vi "5.0.4_HH_Restriction.vi"(6 "Data in":T1, 8 "error in (no error)":errorcluster, 9 "AllControls In":T2, 10 "?":T3, 11 "Message Queue out":T4) -> (0 "error out":errorcluster, 1 "Flow":string, 2 "Data":T3, 3 "Message Queue Out":T4, 4 "Data out":T1)   [LabVIEW 2017]
uses:
  Depends/AMC/subVIs/TypeDefs/amc_Message Queue.ctl
  Depends/AMC/subVIs/TypeDefs/amc_Message.ctl
  Depends/Tools/Keyed Array/Tools_KeyedArray KeyedArray.ctl
  Ctrls/Data.ctl
  Ctrls/AllControls.ctl
  Ctrls/CSV_Data.ctl
  DIPC 692 Daemon API/typdef/get_parameter.ctl
  DIPC 692 Daemon API/typdef/task_detect_test_point.ctl
  DIPC 692 Daemon API/typdef/calibration.ctl
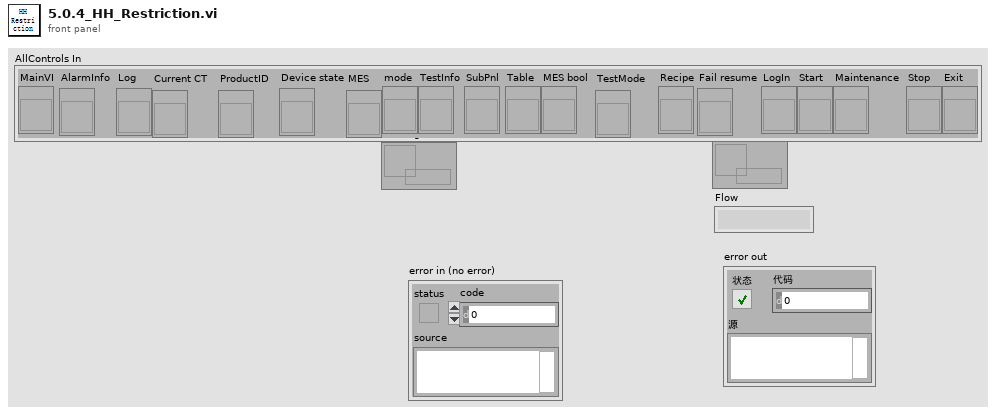
[diagram p1: front panel]
types:
  T1 = typedef "CSV_Data.ctl" = cluster{"Initialisation":cluster{"LMT - Connect UUT (con COM)":string, "LMT - Software Version (rrel)":string, "LMT - Write SKU file (wskuc)":string, "LMT - SKU file name":string, "Connect UUT DDM":string, "Read DDM EOL Timestamp - Mode":string, "Read DDM EOL Timestamp - Timestamp":string, "Read DDM EOL Timestamp - Rig ID":string, "Read DDM EOL Timestamp - Passmark ID":string, "Read DDM EOL Timestamp - Passmark Rev":string, "Software Version before flashing":string, "Read Hardware Serial":string, "UUT DDM SN":string, "Compare DDM SN with MES SN":string, "Backup PCBA Calibration EEPROM Response - CAL":string, "Flash Firmware Version":string, "Check SW Version":string, "Read DDM SW Version after flashing":string, "Set SKU Config":string, "Ready Status":string, "Set Device Mode to EOL":string, "DDM Parameter - Voltage":string, "DDM Parameter - Current":string, "DDM Parameter - Power":string, "DDM Parameter - Speed":string, "DDM Parameter - Pressure":string, "Tester Parameter - Voltage":string, "Tester Parameter - Current":string, "Tester Parameter - Power":string, "Tester Parameter - Ambient Pressure":string, "Tester Parameter - Ambient Temperature":string, "Calculated Parameter - DDM Pressure Corrected":string, "Calculated Parameter - DDM Real Power":string, "Calculated Parameter - Delta V":string}, "BEMF_Calibration":cluster{"Calibration Result - eol_cold_bemf_temp":string, "DDM Ambient Temp":string, "Restriction Plate Diameter":string, "Calibration Result - eol_bemf_mp_cold_coef_a":string, "Calibration Result - eol_bemf_mp_cold_coef_b":string, "Calibration Result - eol_bemf_mp_cold_coef_c":string, "Calibration Result - eol_bemf_lsi_cold_ref_coeffs":string, "Get - Calibration Result - eol_bemf_lsi_speed":string, "Get - Calibration Result - eol_bemf_lsi_integral_0":string, "Calibration Result - eol_bemf_lsi_integral_1":string, "Get - Calibration Result - eol_bemf_lsi_integral_2":string, "Get - Calibration Result - eol_cold_bemf":string, "Get - Calibration Result - eol_cold_bemf_fisf":string, "Finalise Calibration":string, "Compare -Calibration Result - eol_cold_bemf":string, "Compare -Calibration Result - eol_cold_bemf_fisf":string}, "ECO":cluster{"Reset Power Tune":string, "Reset BEMF FISF Calibration":string, "Restriction Plate Diameter":string, "ECO - Stabilisation Time":string, "ECO - DDM Parameter - Voltage":string, "ECO - DDM Parameter - Current":string, "ECO - DDM Parameter - Power":string, "ECO - DDM Parameter - Measured Power":string, "ECO - DDM Parameter - Speed":string, "ECO - DDM Parameter - Pressure":string, "ECO - Tester Parameter - Voltage":string, "ECO - Tester Parameter - Current":string, "ECO - Tester Parameter - Power":string, "ECO - Tester Parameter - Ambient Pressure":string, "ECO - Tester Parameter - Ambient Temperature":string, "ECO - Tester Parameter - Ambient Humidity":string, "ECO - Calculated Parameter - DDM Pressure Corrected":string, "ECO - Calculated Parameter - DDM Real Power":string, "ECO - Calculated Parameter - Delta V":string, "ECO - Calculated Parameter - Flowrate":string, "ECO - Calculated Parameter - Airwatt":string, "ECO - Formula":string, "PT ECO - Power Tune Mode Status":string}, "BOOST":cluster{"Restriction Plate Diameter":string, "BOOST - Stabilisation Time":string, "BOOST - DDM Parameter - Voltage":string, "BOOST - DDM Parameter - Current":string, "BOOST - DDM Parameter - Power":string, "BOOST - DDM Parameter - Measured Power":string, "BOOST - DDM Parameter - Speed":string, "BOOST - DDM Parameter - Pressure":string, "BOOST - Tester Parameter - Voltage":string, "BOOST - Tester Parameter - Current":string, "BOOST - Tester Parameter - Power":string, "BOOST - Tester Parameter - Ambient Pressure":string, "BOOST - Tester Parameter - Ambient Temperature":string, "BOOST - Tester Parameter - Ambient Humidity":string, "BOOST - Calculated Parameter - DDM Pressure Corrected":string, "BOOST - Calculated Parameter - DDM Real Power":string, "BOOST - Calculated Parameter - Delta V":string, "BOOST - Calculated Parameter - Flowrate":string, "BOOST - Calculated Parameter - Airwatt":string, "BOOST - Get AM Presence":string, "Air Muscle Turn Off Status":string, "BOOST - Air Muscle Calculated Parameter - Airwatt B":string, "BOOST - Air Muscle Calculate Airwatt Delta":string, "PT BOOST - Power Tune Mode Status":string, "Finalise Calibration":string, "ECO - Get AW Calibration value":string, "BOOST - Get AW Calibration value":string}, "MAX":cluster{"Restriction Plate Diameter":string, "MAX - Stabilisation Time":string, "Get Average Delta Tmag (LSIdelta_FISFdelta_LSItmag_FISFtmag_IIRtmag)":string, "Get Average Delta Tmag FISF":string, "MAX - DDM Parameter - Voltage":string, "MAX - DDM Parameter - Current":string, "MAX - DDM Parameter - Power":string, "MAX - DDM Parameter - Measured Power":string, "MAX - DDM Parameter - Speed":string, "MAX - DDM Parameter - Pressure":string, "MAX - Tester Parameter - Voltage":string, "MAX - Tester Parameter - Current":string, "MAX - Tester Parameter - Power":string, "MAX - Tester Parameter - Ambient Pressure":string, "MAX - Tester Parameter - Ambient Temperature":string, "MAX - Tester Parameter - Ambient Humidity":string, "MAX - Calculated Parameter - DDM Pressure Corrected":string, "MAX - Calculated Parameter - DDM Real Power":string, "MAX - Calculated Parameter - Delta V":string, "MAX - Calculated Parameter - Flowrate":string, "MAX - Calculated Parameter - Airwatt":string, "MAX_FISF_Check_Average_Delta_Tmag":string, "MAX - FISF - BEMF Finetune Result":string, "MAX tune - Delta P1":string, "MAX tune - Calculated Parameter - Airwatt":string, "Calculate Delta Airwatts - MAX finetune - Delta P2":string, "MAX finetune - DDM Parameter - Voltage":string, "MAX finetune - DDM Parameter - Current":string, "MAX finetune - DDM Parameter - Power":string, "MAX finetune - DDM Parameter - Measured Power":string, "MAX finetune - DDM Parameter - Speed":string, "MAX finetune - DDM Parameter - Pressure":string, "MAX finetune - Tester Parameter - Voltage":string, "MAX finetune - Tester Parameter - Current":string, "MAX finetune - Tester Parameter - Power":string, "MAX finetune - Tester Parameter - Ambient Pressure":string, "MAX finetune - Tester Parameter - Ambient Temperature":string, "MAX finetune - Tester Parameter - Ambient Humidity":string, "MAX finetune - Calculated Parameter - DDM Pressure Corrected":string, "MAX finetune - Calculated Parameter - DDM Real Power":string, "MAX finetune - Calculated Parameter - Delta V":string, "MAX finetune - Calculated Parameter - Flowrate":string, "MAX finetune - Calculated Parameter - Airwatt":string, "Check Derate Result":string, "Delta Tmag FISF":string, "Get Hot BEMF Result":string, "Calculate delta Pressure":string, "Finalise Calibration":string, "Calculate & Check Delta BEMF":string, "Delta P Airwatts Value":string}, "LL":cluster{"DDM Ambient Temp":string, "Restriction Plate Diameter":string, "LL - DDM Parameter - Voltage":string, "LL - DDM Parameter - Current":string, "LL - DDM Parameter - Power":string, "LL - DDM Parameter - Measured Power":string, "LL - DDM Parameter - Speed":string, "LL - DDM Parameter - Pressure":string, "LL - Tester Parameter - Voltage":string, "LL - Tester Parameter - Current":string, "LL - Tester Parameter - Power":string, "LL - DDM Real Power":string, "LL - Calibrate Task Detect LL":string}, "HL":cluster{"HL - DDM Parameter - Voltage":string, "HL - DDM Parameter - Current":string, "HL - DDM Parameter - Power":string, "HL - DDM Parameter - Measured Power":string, "HL - DDM Parameter - Speed":string, "HL - DDM Parameter - Pressure":string, "HL - Tester Parameter - Voltage":string, "HL - Tester Parameter - Current":string, "HL - Tester Parameter - Power":string, "HL - DDM Real Power":string, "HL - Calibrate Task Detect HL":string}, "LH":cluster{"Restriction Plate Diameter":string, "LH - DDM Parameter - Voltage":string, "LH - DDM Parameter - Current":string, "LH - DDM Parameter - Power":string, "LH - DDM Parameter - Measured Power":string, "LH - DDM Parameter - Speed":string, "LH - DDM Parameter - Pressure":string, "LH - Tester Parameter - Voltage":string, "LH - Tester Parameter - Current":string, "LH - Tester Parameter - Power":string, "LH - DDM Real Power":string, "LH - Calibrate Task Detect LH":string}, "HH":cluster{"HH - DDM Parameter - Voltage":string, "HH - DDM Parameter - Current":string, "HH - DDM Parameter - Power":string, "HH - DDM Parameter - Measured Power":string, "HH - DDM Parameter - Speed":string, "HH - DDM Parameter - Pressure":string, "HH - Tester Parameter - Voltage":string, "HH - Tester Parameter - Current":string, "HH - Tester Parameter - Power":string, "HH - DDM Real Power":string, "HH - Calibrate Task Detect HH":string}, "Inlet Blockage Calibration":cluster{"Inlet Blockage Calibration - DDM Parameter - Voltage":string, "Inlet Blockage Calibration - DDM Parameter - Current":string, "Inlet Blockage Calibration - DDM Parameter - Power":string, "Inlet Blockage Calibration - DDM Parameter - Measured Power":string, "Inlet Blockage Calibration - DDM Parameter - Speed":string, "Inlet Blockage Calibration - DDM Parameter - Pressure":string, "Inlet Blockage Calibration - Tester Parameter - Voltage":string, "Inlet Blockage Calibration - Tester Parameter - Current":string, "Inlet Blockage Calibration - Tester Parameter - Power":string, "Inlet Blockage Calibration - DDM Real Power":string, "Calibration Inlet Blockage_E":string, "Finalise Calibration":string, "Get Task Detect LL":string, "Get Task Detect HL":string, "Get Task Detect LH":string, "Get Task Detect HH":string, "Calibration Inlet Blockage":string, "Calibration eol cold bemf temp":string}, "GOOD":cluster{"GOOD UNIT - Clear EEPROM Error Log":string, "GOOD UNIT - Write Product Timestamp - Mode":string, "GOOD UNIT - Write Product Timestamp - Timestamp":string, "GOOD UNIT - Write Product Timestamp - Rig ID":string, "GOOD UNIT - Write Product Timestamp - Passmark ID":string, "GOOD UNIT - Write Product Timestamp - Passmark Rev":string, "GOOD UNIT - Set Device Mode to PROD":string, "GOOD UNIT - Backup PCBA Calibration EEPROM Response":string, "GOOD UNIT - Check Security Bit":string, "GOOD UNIT - Set Calibration Lock":string, "GOOD UNIT - Get_Calibration_Lock":string, "GOOD UNIT - Disconnect UUT":string}, "NG":cluster{"NG UNIT - Read NVM Error":string, "NG UNIT - Set Device Mode to FCT":string, "NG UNIT - Backup PCBA Calibration EEPROM Response - CAL":string, "NG UNIT - Backup PCBA Calibration EEPROM Response - ERROR":string, "NG UNIT - Backup PCBA Calibration EEPROM Response - USAGE":string, "NG UNIT - Disconnect UUT":string}, "SN":string, "Table":string[][], "Count":cluster{"Total":i32, "OK":i32, "NG":i32, "Yield":dbl}, "Start Time":timestamp, "daemon reference":refnum<k5>, "CT":dbl, "Config":string[][], "OK/NG":bool, "Station ID":string, "MES DDM SN":string, "MES PCBA SN":string, "Retest":string, "Lux":string, "Initialisation_Status":cluster{"LMT - Connect UUT (con COM)":string, "LMT - Software Version (rrel)":string, "LMT - Write SKU file (wskuc)":string, "LMT - SKU file name":string, "Connect UUT DDM":string, "Read DDM EOL Timestamp - Mode":string, "Read DDM EOL Timestamp - Timestamp":string, "Read DDM EOL Timestamp - Rig ID":string, "Read DDM EOL Timestamp - Passmark ID":string, "Read DDM EOL Timestamp - Passmark Rev":string, "Software Version before flashing":string, "Read Hardware Serial":string, "UUT DDM SN":string, "Compare DDM SN with MES SN":string, "Backup PCBA Calibration EEPROM Response - CAL":string, "Flash Firmware Version":string, "Check SW Version":string, "Read DDM SW Version after flashing":string, "Set SKU Config":string, "Ready Status":string, "Set Device Mode to EOL":string, "DDM Parameter - Voltage":string, "DDM Parameter - Current":string, "DDM Parameter - Power":string, "DDM Parameter - Speed":string, "DDM Parameter - Pressure":string, "Tester Parameter - Voltage":string, "Tester Parameter - Current":string, "Tester Parameter - Power":string, "Tester Parameter - Ambient Pressure":string, "Tester Parameter - Ambient Temperature":string, "Calculated Parameter - DDM Pressure Corrected":string, "Calculated Parameter - DDM Real Power":string, "Calculated Parameter - Delta V":string}, "BEMF_Calibration_Status":cluster{"Calibration Result - eol_cold_bemf_temp":string, "DDM Ambient Temp":string, "Restriction Plate Diameter":string, "Calibration Result - eol_bemf_mp_cold_coef_a":string, "Calibration Result - eol_bemf_mp_cold_coef_b":string, "Calibration Result - eol_bemf_mp_cold_coef_c":string, "Calibration Result - eol_bemf_lsi_cold_ref_coeffs":string, "Get - Calibration Result - eol_bemf_lsi_speed":string, "Get - Calibration Result - eol_bemf_lsi_integral_0":string, "Calibration Result - eol_bemf_lsi_integral_1":string, "Get - Calibration Result - eol_bemf_lsi_integral_2":string, "Get - Calibration Result - eol_cold_bemf":string, "Get - Calibration Result - eol_cold_bemf_fisf":string, "Finalise Calibration":string, "Compare -Calibration Result - eol_cold_bemf":string, "Compare -Calibration Result - eol_cold_bemf_fisf":string}, "ECO_Status":cluster{"Reset Power Tune":string, "Reset BEMF FISF Calibration":string, "Restriction Plate Diameter":string, "ECO - Stabilisation Time":string, "ECO - DDM Parameter - Voltage":string, "ECO - DDM Parameter - Current":string, "ECO - DDM Parameter - Power":string, "ECO - DDM Parameter - Measured Power":string, "ECO - DDM Parameter - Speed":string, "ECO - DDM Parameter - Pressure":string, "ECO - Tester Parameter - Voltage":string, "ECO - Tester Parameter - Current":string, "ECO - Tester Parameter - Power":string, "ECO - Tester Parameter - Ambient Pressure":string, "ECO - Tester Parameter - Ambient Temperature":string, "ECO - Tester Parameter - Ambient Humidity":string, "ECO - Calculated Parameter - DDM Pressure Corrected":string, "ECO - Calculated Parameter - DDM Real Power":string, "ECO - Calculated Parameter - Delta V":string, "ECO - Calculated Parameter - Flowrate":string, "ECO - Calculated Parameter - Airwatt":string, "ECO - Formula":string, "PT ECO - Power Tune Mode Status":string}, "BOOST_Status":cluster{"Restriction Plate Diameter":string, "BOOST - Stabilisation Time":string, "BOOST - DDM Parameter - Voltage":string, "BOOST - DDM Parameter - Current":string, "BOOST - DDM Parameter - Power":string, "BOOST - DDM Parameter - Measured Power":string, "BOOST - DDM Parameter - Speed":string, "BOOST - DDM Parameter - Pressure":string, "BOOST - Tester Parameter - Voltage":string, "BOOST - Tester Parameter - Current":string, "BOOST - Tester Parameter - Power":string, "BOOST - Tester Parameter - Ambient Pressure":string, "BOOST - Tester Parameter - Ambient Temperature":string, "BOOST - Tester Parameter - Ambient Humidity":string, "BOOST - Calculated Parameter - DDM Pressure Corrected":string, "BOOST - Calculated Parameter - DDM Real Power":string, "BOOST - Calculated Parameter - Delta V":string, "BOOST - Calculated Parameter - Flowrate":string, "BOOST - Calculated Parameter - Airwatt":string, "BOOST - Get AM Presence":string, "Air Muscle Turn Off Status":string, "BOOST - Air Muscle Calculated Parameter - Airwatt B":string, "BOOST - Air Muscle Calculate Airwatt Delta":string, "PT BOOST - Power Tune Mode Status":string, "Finalise Calibration":string, "ECO - Get AW Calibration value":string, "BOOST - Get AW Calibration value":string}, "MAX_Status":cluster{"Restriction Plate Diameter":string, "MAX - Stabilisation Time":string, "Get Average Delta Tmag (LSIdelta_FISFdelta_LSItmag_FISFtmag_IIRtmag)":string, "Get Average Delta Tmag FISF":string, "MAX - DDM Parameter - Voltage":string, "MAX - DDM Parameter - Current":string, "MAX - DDM Parameter - Power":string, "MAX - DDM Parameter - Measured Power":string, "MAX - DDM Parameter - Speed":string, "MAX - DDM Parameter - Pressure":string, "MAX - Tester Parameter - Voltage":string, "MAX - Tester Parameter - Current":string, "MAX - Tester Parameter - Power":string, "MAX - Tester Parameter - Ambient Pressure":string, "MAX - Tester Parameter - Ambient Temperature":string, "MAX - Tester Parameter - Ambient Humidity":string, "MAX - Calculated Parameter - DDM Pressure Corrected":string, "MAX - Calculated Parameter - DDM Real Power":string, "MAX - Calculated Parameter - Delta V":string, "MAX - Calculated Parameter - Flowrate":string, "MAX - Calculated Parameter - Airwatt":string, "MAX_FISF_Check_Average_Delta_Tmag":string, "MAX - FISF - BEMF Finetune Result":string, "MAX tune - Delta P1":string, "MAX tune - Calculated Parameter - Airwatt":string, "Calculate Delta Airwatts - MAX finetune - Delta P2":string, "MAX finetune - DDM Parameter - Voltage":string, "MAX finetune - DDM Parameter - Current":string, "MAX finetune - DDM Parameter - Power":string, "MAX finetune - DDM Parameter - Measured Power":string, "MAX finetune - DDM Parameter - Speed":string, "MAX finetune - DDM Parameter - Pressure":string, "MAX finetune - Tester Parameter - Voltage":string, "MAX finetune - Tester Parameter - Current":string, "MAX finetune - Tester Parameter - Power":string, "MAX finetune - Tester Parameter - Ambient Pressure":string, "MAX finetune - Tester Parameter - Ambient Temperature":string, "MAX finetune - Tester Parameter - Ambient Humidity":string, "MAX finetune - Calculated Parameter - DDM Pressure Corrected":string, "MAX finetune - Calculated Parameter - DDM Real Power":string, "MAX finetune - Calculated Parameter - Delta V":string, "MAX finetune - Calculated Parameter - Flowrate":string, "MAX finetune - Calculated Parameter - Airwatt":string, "Check Derate Result":string, "Delta Tmag FISF":string, "Get Hot BEMF Result":string, "Calculate delta Pressure":string, "Finalise Calibration":string, "Calculate & Check Delta BEMF":string, "Delta P Airwatts Value":string}, "LL_Status":cluster{"DDM Ambient Temp":string, "Restriction Plate Diameter":string, "LL - DDM Parameter - Voltage":string, "LL - DDM Parameter - Current":string, "LL - DDM Parameter - Power":string, "LL - DDM Parameter - Measured Power":string, "LL - DDM Parameter - Speed":string, "LL - DDM Parameter - Pressure":string, "LL - Tester Parameter - Voltage":string, "LL - Tester Parameter - Current":string, "LL - Tester Parameter - Power":string, "LL - DDM Real Power":string, "LL - Calibrate Task Detect LL":string}, "HL_Status":cluster{"HL - DDM Parameter - Voltage":string, "HL - DDM Parameter - Current":string, "HL - DDM Parameter - Power":string, "HL - DDM Parameter - Measured Power":string, "HL - DDM Parameter - Speed":string, "HL - DDM Parameter - Pressure":string, "HL - Tester Parameter - Voltage":string, "HL - Tester Parameter - Current":string, "HL - Tester Parameter - Power":string, "HL - DDM Real Power":string, "HL - Calibrate Task Detect HL":string}, "LH_Status":cluster{"Restriction Plate Diameter":string, "LH - DDM Parameter - Voltage":string, "LH - DDM Parameter - Current":string, "LH - DDM Parameter - Power":string, "LH - DDM Parameter - Measured Power":string, "LH - DDM Parameter - Speed":string, "LH - DDM Parameter - Pressure":string, "LH - Tester Parameter - Voltage":string, "LH - Tester Parameter - Current":string, "LH - Tester Parameter - Power":string, "LH - DDM Real Power":string, "LH - Calibrate Task Detect LH":string}, "HH_Status":cluster{"HH - DDM Parameter - Voltage":string, "HH - DDM Parameter - Current":string, "HH - DDM Parameter - Power":string, "HH - DDM Parameter - Measured Power":string, "HH - DDM Parameter - Speed":string, "HH - DDM Parameter - Pressure":string, "HH - Tester Parameter - Voltage":string, "HH - Tester Parameter - Current":string, "HH - Tester Parameter - Power":string, "HH - DDM Real Power":string, "HH - Calibrate Task Detect HH":string}, "Inlet Blockage Calibration_Status":cluster{"Inlet Blockage Calibration - DDM Parameter - Voltage":string, "Inlet Blockage Calibration - DDM Parameter - Current":string, "Inlet Blockage Calibration - DDM Parameter - Power":string, "Inlet Blockage Calibration - DDM Parameter - Measured Power":string, "Inlet Blockage Calibration - DDM Parameter - Speed":string, "Inlet Blockage Calibration - DDM Parameter - Pressure":string, "Inlet Blockage Calibration - Tester Parameter - Voltage":string, "Inlet Blockage Calibration - Tester Parameter - Current":string, "Inlet Blockage Calibration - Tester Parameter - Power":string, "Inlet Blockage Calibration - DDM Real Power":string, "Calibration Inlet Blockage_E":string, "Finalise Calibration":string, "Get Task Detect LL":string, "Get Task Detect HL":string, "Get Task Detect LH":string, "Get Task Detect HH":string, "Calibration Inlet Blockage":string, "Calibration eol cold bemf temp":string}, "GOOD_Status":cluster{"GOOD UNIT - Clear EEPROM Error Log":string, "GOOD UNIT - Write Product Timestamp - Mode":string, "GOOD UNIT - Write Product Timestamp - Timestamp":string, "GOOD UNIT - Write Product Timestamp - Rig ID":string, "GOOD UNIT - Write Product Timestamp - Passmark ID":string, "GOOD UNIT - Write Product Timestamp - Passmark Rev":string, "GOOD UNIT - Set Device Mode to PROD":string, "GOOD UNIT - Backup PCBA Calibration EEPROM Response":string, "GOOD UNIT - Check Security Bit":string, "GOOD UNIT - Set Calibration Lock":string, "GOOD UNIT - Get_Calibration_Lock":string, "GOOD UNIT - Disconnect UUT":string}, "NG_Status":cluster{"NG UNIT - Read NVM Error":string, "NG UNIT - Set Device Mode to FCT":string, "NG UNIT - Backup PCBA Calibration EEPROM Response - CAL":string, "NG UNIT - Backup PCBA Calibration EEPROM Response - ERROR":string, "NG UNIT - Backup PCBA Calibration EEPROM Response - USAGE":string, "NG UNIT - Disconnect UUT":string}, "SKU":string, "Plate_Diameter":string, "Alarm":string}
  T2 = typedef "AllControls.ctl" = cluster{"MainVI":refnum<vi>, "AlarmInfo":refnum<vi>, "Log":refnum<vi>, "Current CT":refnum<vi>, "ProductID":refnum<vi>, "Device state":refnum<vi>, "MES":refnum<vi>, "mode":refnum<vi>, "TestInfo":refnum<vi>, "SubPnl":refnum<vi>, "Table":refnum<vi>, "MES bool":refnum<vi>, "TestMode":refnum<vi>, "Recipe":refnum<vi>, "Fail resume":refnum<vi>, "LogIn":refnum<vi>, "Start":refnum<vi>, "Maintenance":refnum<vi>, "Stop":refnum<vi>, "Exit":refnum<vi>}
  T3 = typedef "Data.ctl" = cluster{"Initialisation":cluster{"DDM_Parameter":dbl[], "DDM_Parameter_status":bool[], "Get_Tester_Parameter":dbl[], "Get_Tester_Parameter_status":bool[], "Cal_Tester_Parameter":dbl[], "Cal_Tester_Parameter_status":bool[], "sw_version_before_status":bool, "sw_version_after_status":bool, "Set_SKU_Config_With_LMT_status":bool, "FCT_timestamp_status":bool, "LMT_Connect_to_UUT_status":bool}, "BEMF_Calibration":cluster{"Read_ambient_temperature":dbl, "Calibration_Vaule":dbl[], "Calibration_Vaule _B":dbl[], "Calibration_Vaule_status":bool[], "Calibration_Vaule_B_status":bool[]}, "ECO":cluster{"DDM_Parameter":dbl[], "DDM_Parameter_status":bool[], "Get_Tester_Parameter":dbl[], "Get_Tester_Parameter_status":bool[], "Cal_Tester_Parameter":dbl[], "Cal_Tester_Parameter_status":bool[], "DDM_Parameter_after_power_tune":dbl[], "Get_Tester_Parameter_after_power_tune":dbl[], "Cal_Tester_Parameter_after_power_tune":dbl[], "Cal_Tester_Parameter_after_power_tune_status":bool[], "Delta_P":dbl}, "BOOST":cluster{"DDM_Parameter":dbl[], "DDM_Parameter_status":bool[], "Get_Tester_Parameter":dbl[], "Get_Tester_Parameter_status":bool[], "Cal_Tester_Parameter":dbl[], "Cal_Tester_Parameter_status":bool[], "DDM_Parameter_after_power_tune":dbl[], "Get_Tester_Parameter_after_power_tune":dbl[], "Cal_Tester_Parameter_after_power_tune":dbl[], "Cal_Tester_Parameter_after_power_tune_status":bool[], "airwatts_am_off":dbl, "AW_Delta_(AM_on_and_off)":dbl, "AW_Delta_(AM_on_and_off)_Status":bool, "Delta_P":dbl}, "MAX":cluster{"Average_Tmag_Data":cluster{"LSI Delta in degC":dbl, "FISF Delta in degc":dbl, "LSI Tmag in degC":dbl, "Fisf Tmag in degC":dbl, "IIR Tmag in degC":dbl}, "DDM_Parameter":dbl[], "DDM_Parameter_status":bool[], "Get_Tester_Parameter":dbl[], "Get_Tester_Parameter_status":bool[], "Cal_Tester_Parameter":dbl[], "BEMF_Finetune":cluster{"eol_bemf_mp_cold_coef_c":dbl, "eol_cold_bemf_fisf_offset":dbl}, "AW_Tune":cluster{"delta_P1":dbl, "delta_P_Setting":dbl}, "DDM_Parameter_after_Airwatts_Tune":dbl[], "Get_Tester_Parameter_after_Airwatts_Tune":dbl[], "Cal_Tester_Parameter_after_Airwatts_Tune":dbl[], "DDM_Parameter_after_Airwatts_Finetune":dbl[], "Get_Tester_Parameter_after_Airwatts_Finetune":dbl[], "Cal_Tester_Parameter_after_Airwatts_Finetune":dbl[], "AW_Finetune":cluster{"delta_P2":dbl, "delta_P_Setting":dbl}, "Delta_Tmag_after_tune":cluster{"LSI Delta in degC":dbl, "FISF Delta in degc":dbl, "LSI Tmag in degC":dbl, "Fisf Tmag in degC":dbl, "IIR Tmag in degC":dbl}, "Hot Bemf in mV":dbl, "DDM_Pressure":dbl, "Delta_Pressure":dbl, " Cold Bemf in mV":dbl, " delta Bemf":dbl, " delta p":dbl, "Delta_Pressure_status":bool, " delta Bemf_status":bool, "LSI Delta in degC_status":bool, "FISF Delta in degc_status":bool, "Max_check_derate_status_status":bool, "Average_All_data":dbl[][], "Average_Tmag_Data_status":bool[], "Average_Tmag_Data_after_tune_status":bool[], "Cal_Tester_Parameter_status":bool[], "Cal_Tester_Parameter_status_after_Airwatts_Tune":bool[], "Cal_Tester_Parameter_status_after_Airwatts_FineTune":bool[]}, "Task_Detect_Calib":cluster{"LL":cluster{"DDM_Parameter":dbl[], "DDM_Parameter_status":bool[], "Get_Tester_Parameter":dbl[], "Get_Tester_Parameter_status":bool[], "Set_task_detect_A":dbl, "Set_task_detect_A_Status":bool}, "HL":cluster{"DDM_Parameter":dbl[], "DDM_Parameter_status":bool[], "Get_Tester_Parameter":dbl[], "Get_Tester_Parameter_status":bool[], "Set_task_detect_B":dbl, "Set_task_detect_B_Status":bool}, "LH":cluster{"DDM_Parameter":dbl[], "DDM_Parameter_status":bool[], "Get_Tester_Parameter":dbl[], "Get_Tester_Parameter_status":bool[], "Set_task_detect_C":dbl, "Set_task_detect_C_Status":bool}, "HH":cluster{"DDM_Parameter":dbl[], "DDM_Parameter_status":bool[], "Get_Tester_Parameter":dbl[], "Get_Tester_Parameter_status":bool[], "Set_task_detect_D":dbl, "Read_and_check_calibration_Status":bool[], "Set_task_detect_D_Status":bool}, "Get_eol_inlet_blockage_E":dbl, "Calib_vaule":cluster{"Get_task_detect_LL":dbl, "Get_task_detect_HL":dbl, "Get_task_detect_LH":dbl, "Get_task_detect_HH":dbl, "eol_inlet_blockage":dbl, "eol_code_bemf_temp":dbl}, "calibrated temp":dbl, "Inlet_Blockage_Calibration":cluster{"DDM_Parameter":dbl[], "DDM_Parameter_status":bool[], "Get_Tester_Parameter":dbl[], "Get_Tester_Parameter_status":bool[]}, "Get_eol_inlet_blockage_E_Status":bool}, "good":cluster{"Write_Product_TS":cluster{"TIMESTAMP":i64, "RIG_ID":i64, "PASSMARK_ID":i64, "PASSMARK_REV":i64}, "Read_Product_TS":cluster{"TIMESTAMP":i64, "RIG_ID":i64, "PASSMARK_ID":i64, "PASSMARK_REV":i64}, "Good_Check_Secuity_Bit_Stauts":bool}}
  T4 = typedef "amc_Message Queue.ctl" = refnum<queue>
  T5 = typedef "HD Config.ctl" = cluster{" PC":cluster{"PC Address":u8[], "PC Port":i32}, "FCO":cluster{"COM":refnum<visa-resource-name>, "Baudrate":u32}, "DC Power ":cluster{"COM":refnum<visa-resource-name>, "Baudrate":u32}, "PW3336":cluster{"COM":refnum<visa-resource-name>, "Baudrate":u32}, "Lefoo":cluster{"COM":refnum<visa-resource-name>, "Baudrate":u32}, "Tempt&Hum":cluster{"COM":refnum<visa-resource-name>, "Baudrate":u32}, "DIPC":cluster{"COM":refnum<visa-resource-name>}, "Daemon":cluster{"IP Address":string, "Port":u16, "Retry":u16}, "NFC":cluster{"COM":refnum<visa-resource-name>, "Baudrate":u32}, "Fail_resume_mode":bool, "GRR":bool}
  T6 = typedef "get_parameter.ctl" = string
  T7 = typedef "task_detect_test_point.ctl" = enum16{"LL", "HL", "LH", "HH"}
  T8 = typedef "calibration.ctl" = string
  T9 = cluster{"[0]":dbl, "[1]":dbl, "[2]":dbl, "[3]":dbl, "[4]":dbl, "[5]":dbl}
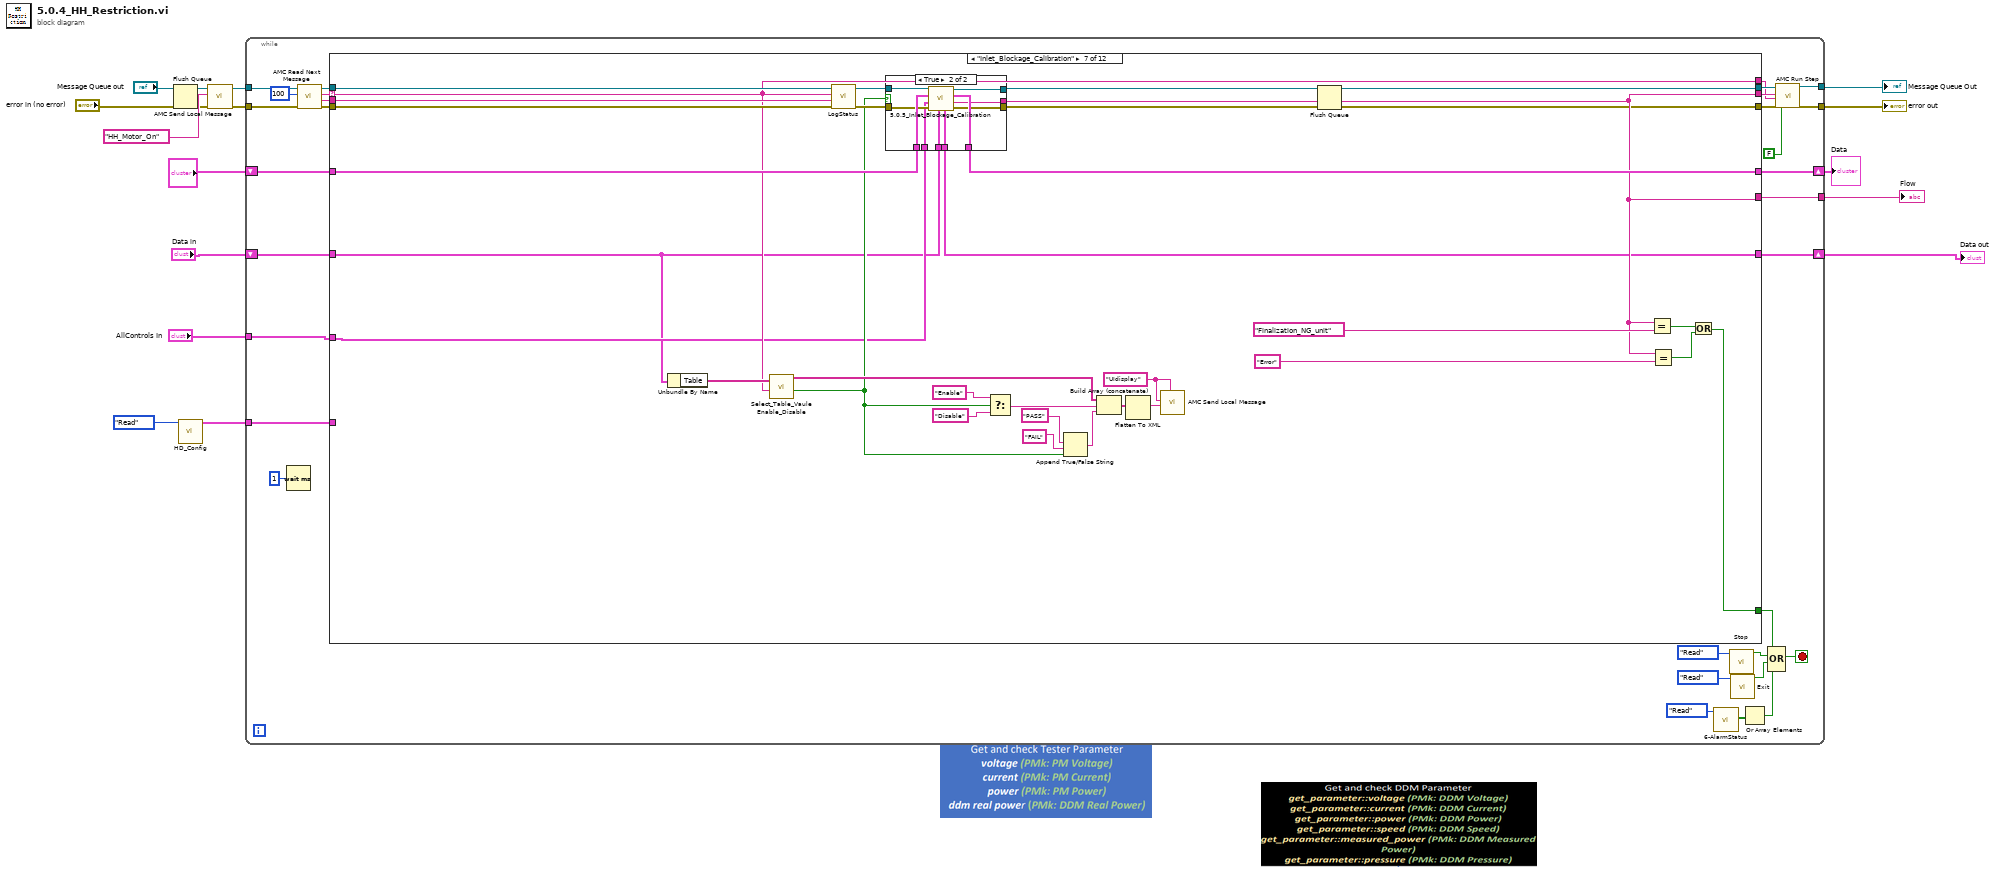
[diagram p0: block diagram]
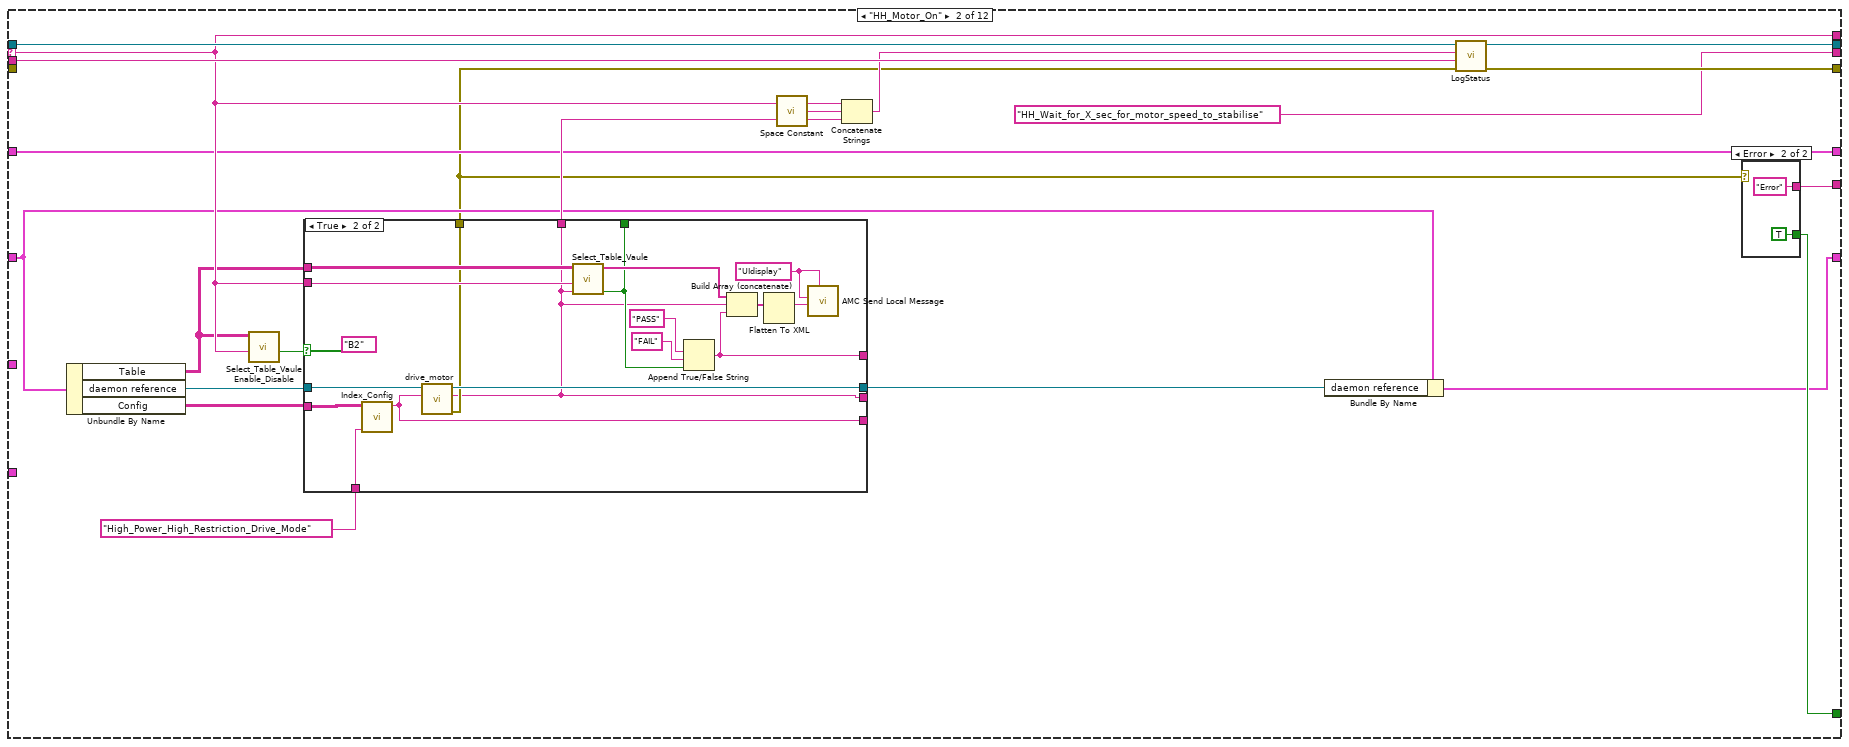
[diagram p3: hidden frame]
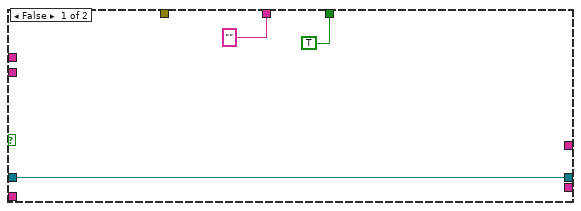
[diagram p5: hidden frame]
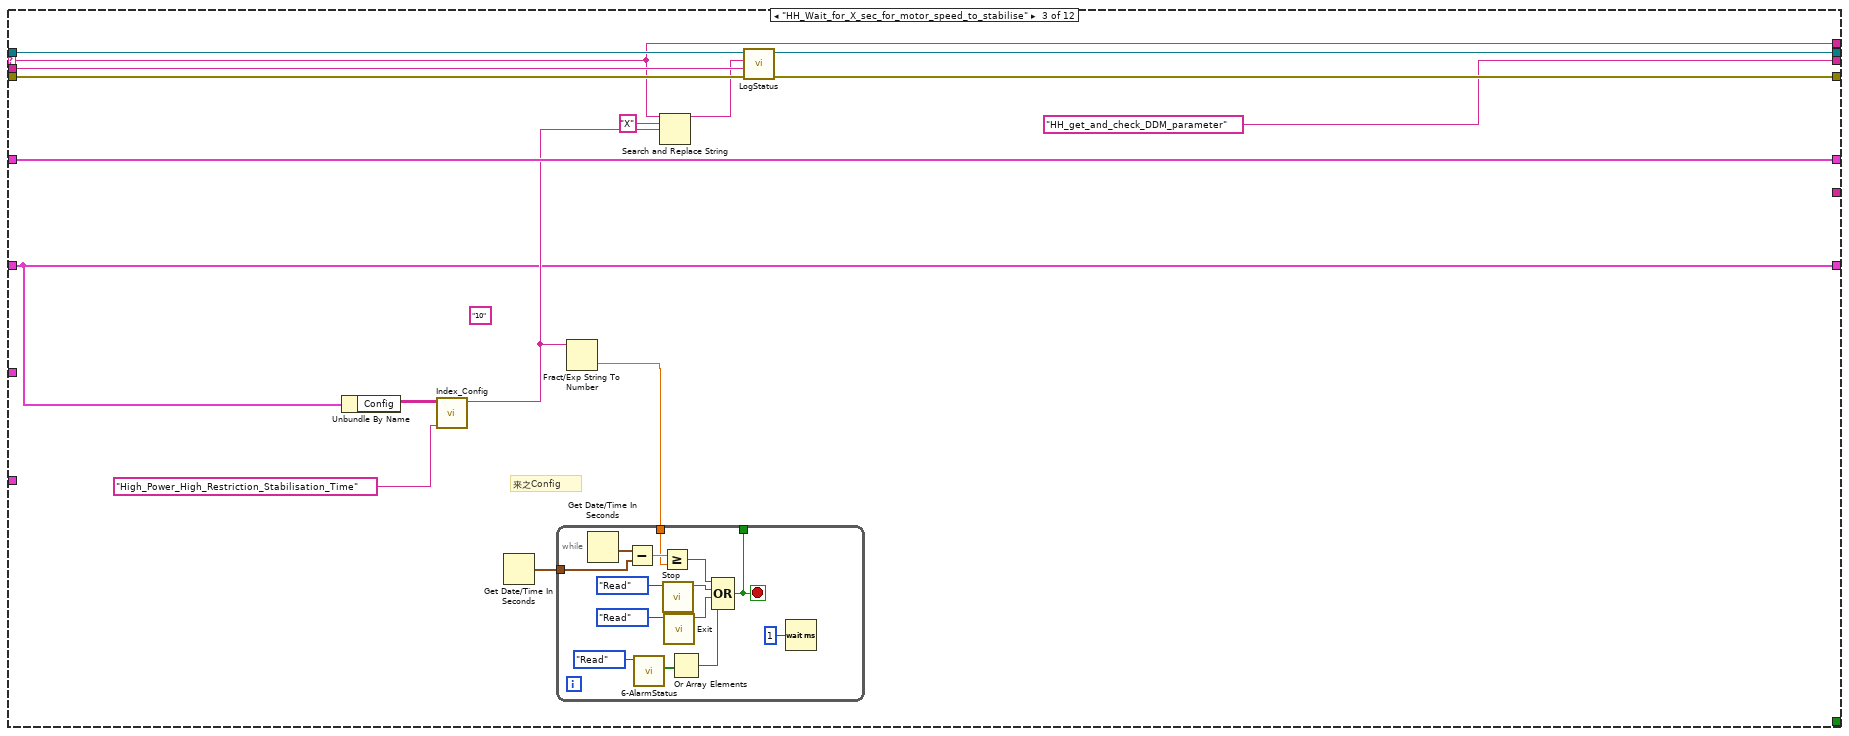
[diagram p6: hidden frame]
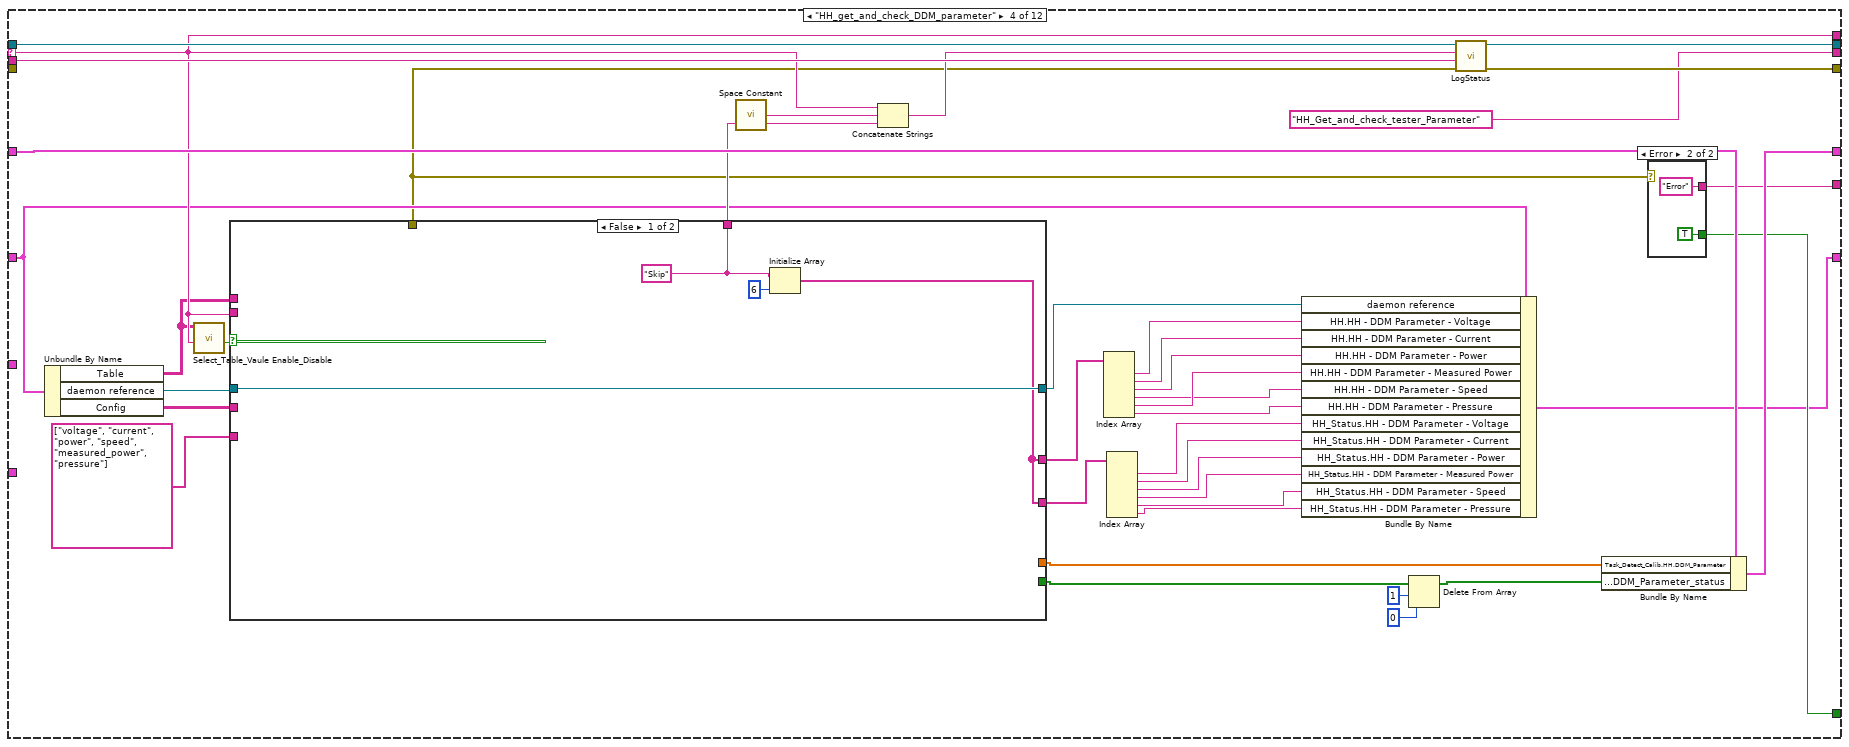
[diagram p7: hidden frame]
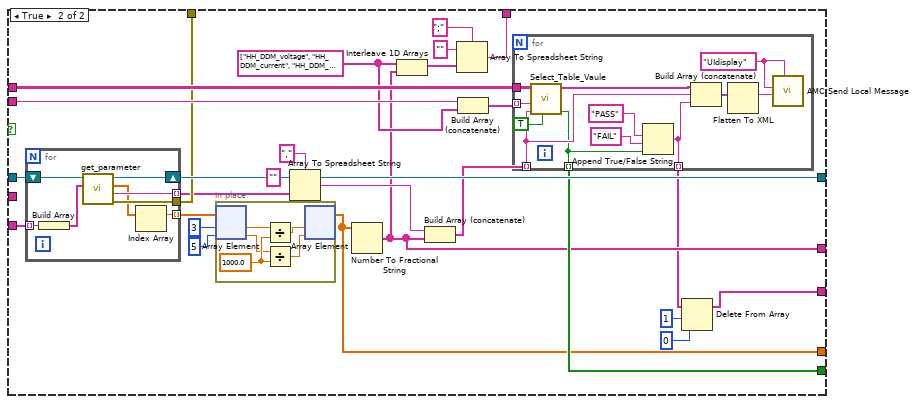
[diagram p9: hidden frame]
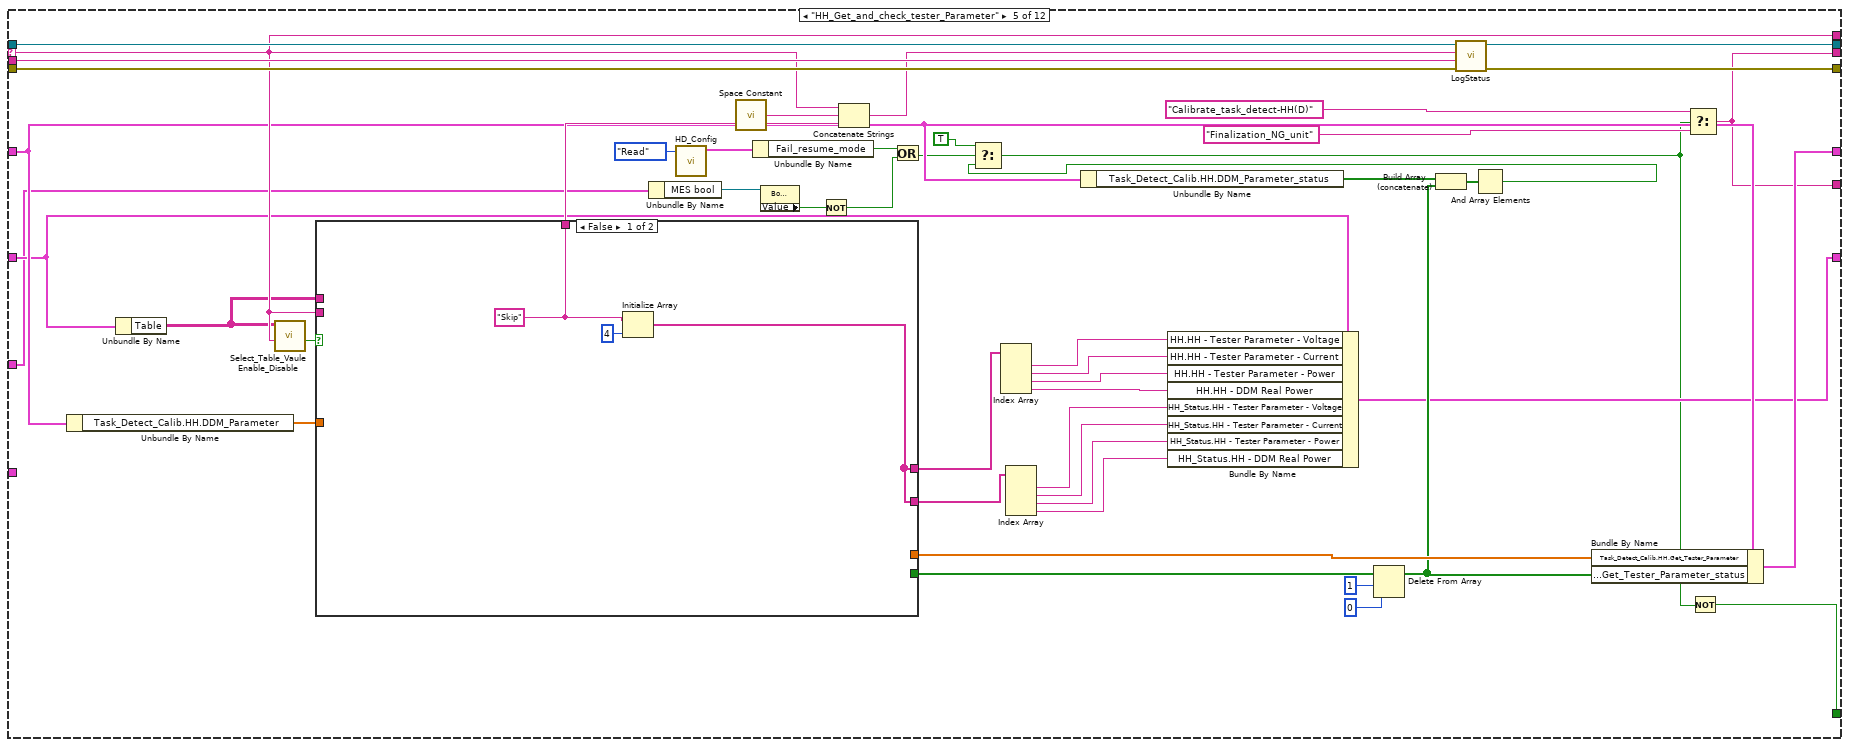
[diagram p10: hidden frame]
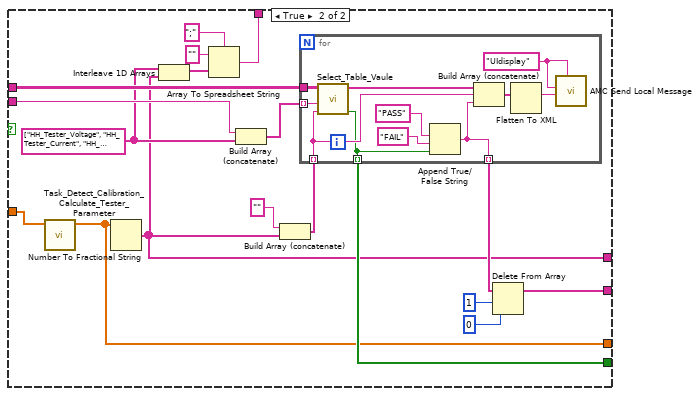
[diagram p11: hidden frame]
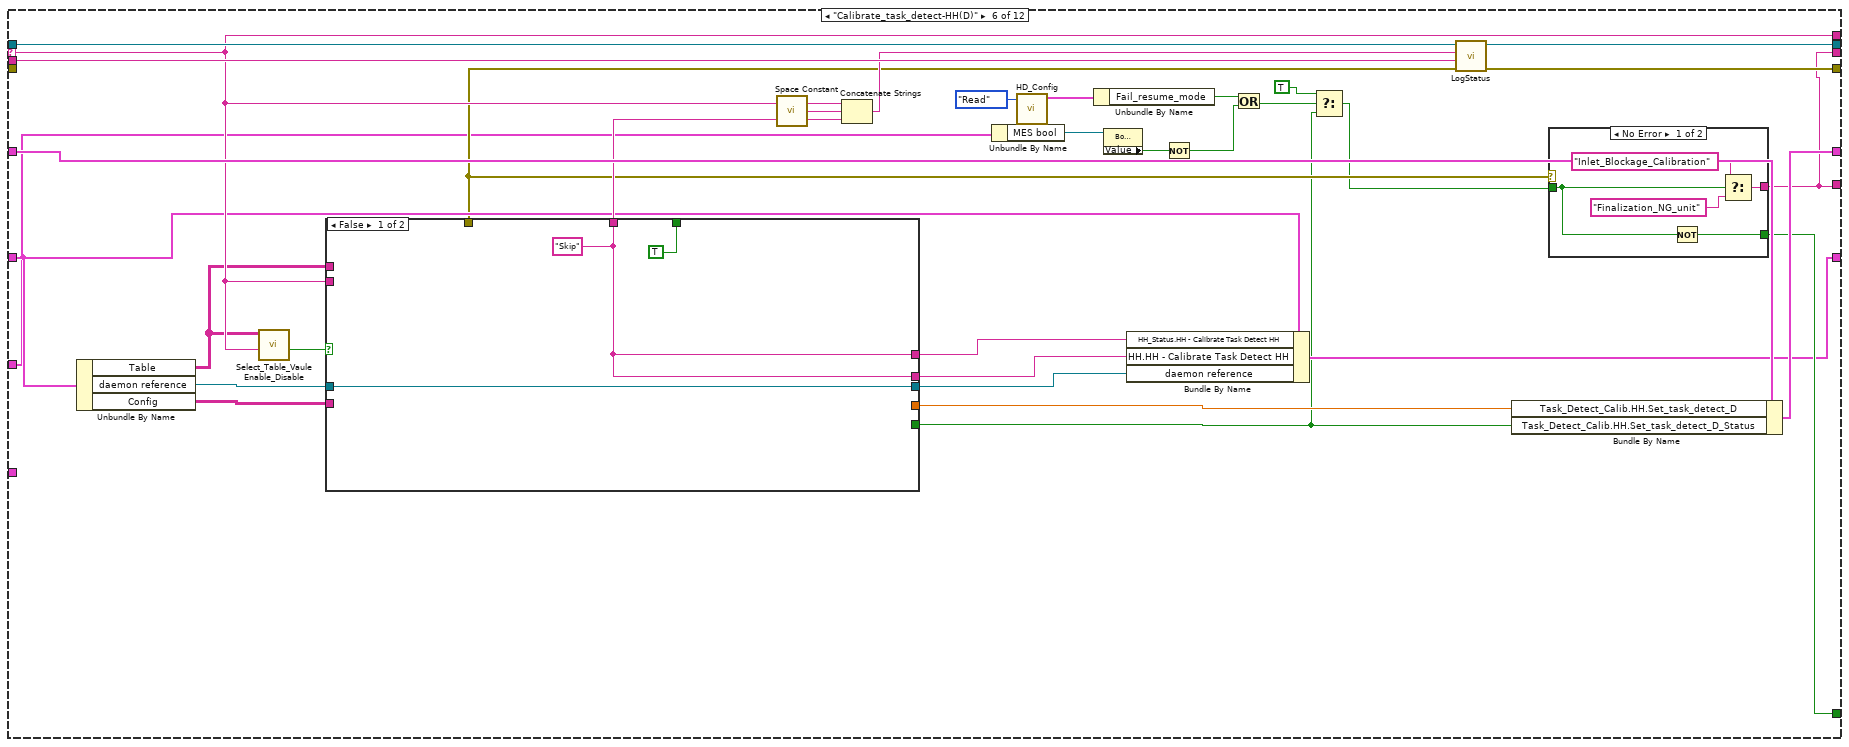
[diagram p12: hidden frame]
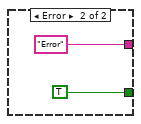
[diagram p13: hidden frame]
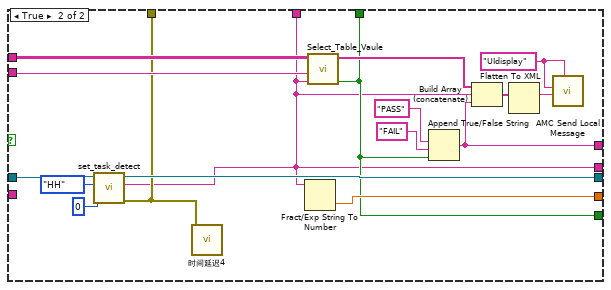
[diagram p14: hidden frame]
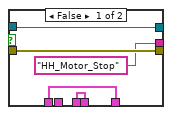
[diagram p15: hidden frame]
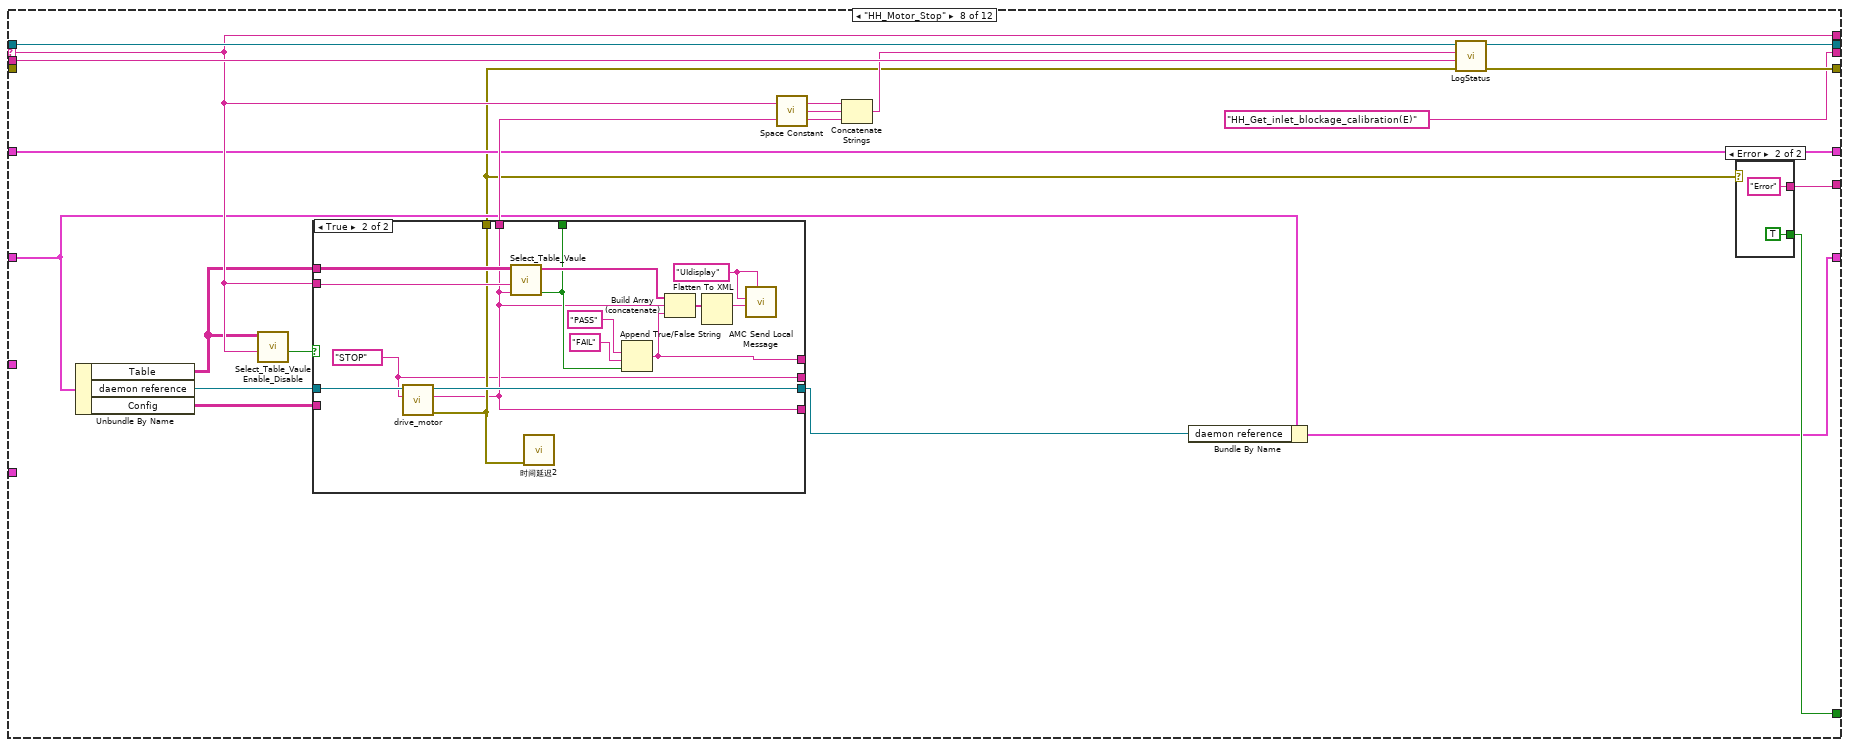
[diagram p16: hidden frame]
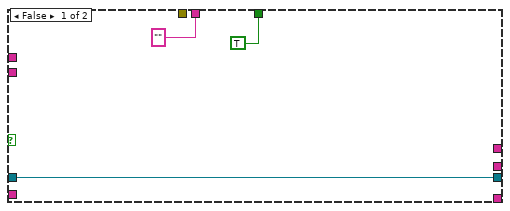
[diagram p18: hidden frame]
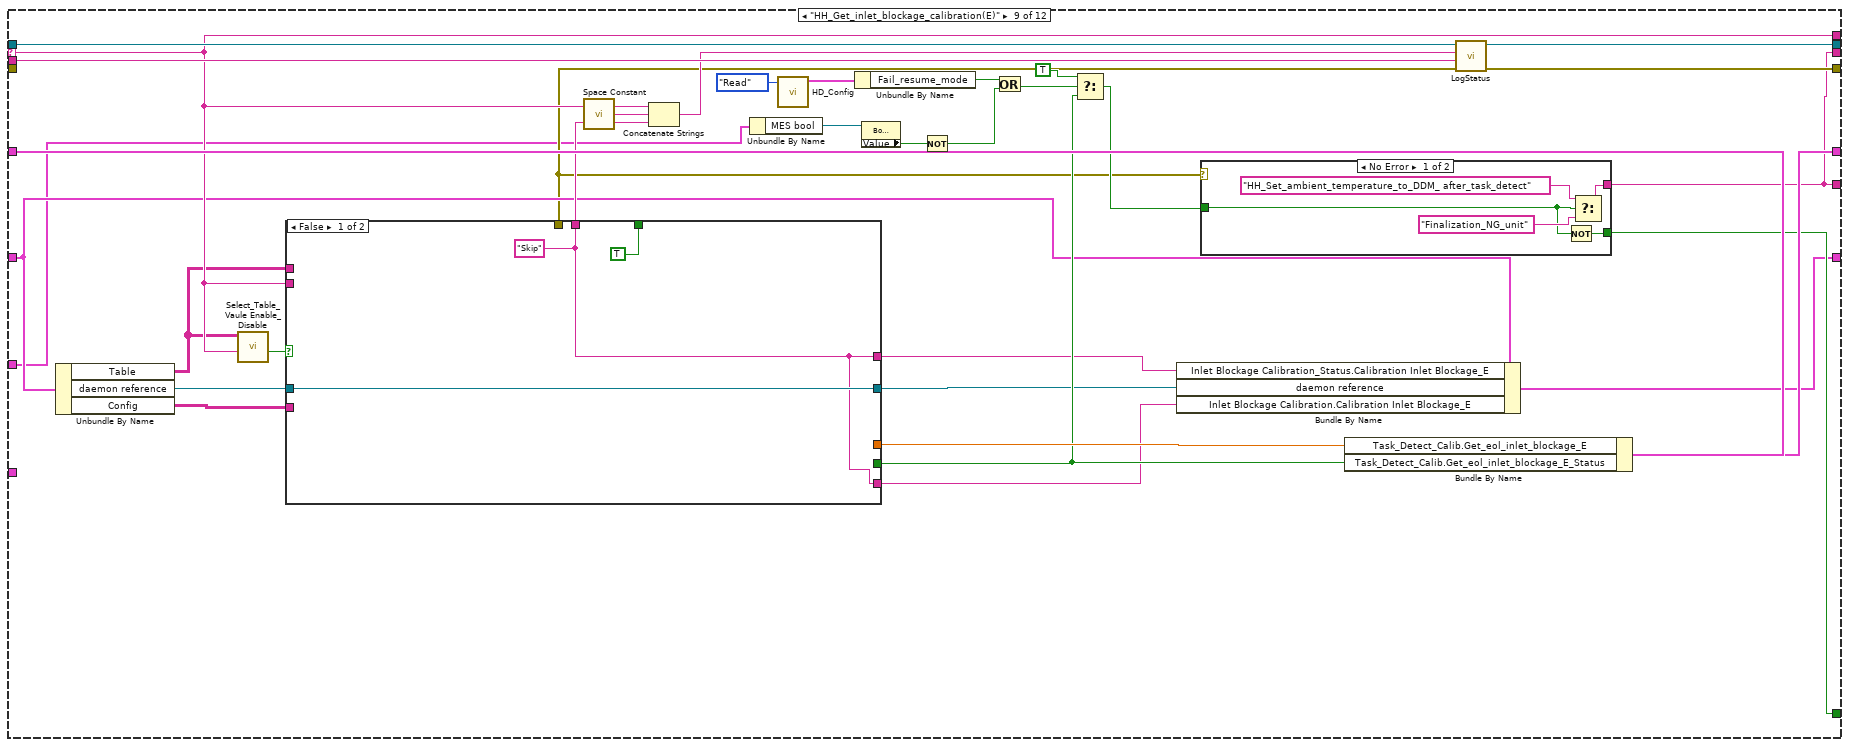
[diagram p19: hidden frame]
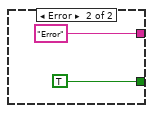
[diagram p20: hidden frame]
diagram:
  n1 = Flush Queue(queue="Message Queue out") -> (queue out=w4:T4)  [unwired: 1 in, 2 out]
  n2 = call "HD_Config.vi"("Step"=enum16{"Initial", "Write", "Read"}."Read") -> ("HD Config out"=w8:T5)  [unwired: 9 in, 1 out]
  n3 = call "AMC Send Local Message.vi"("error in (no error)"="error in (no error)", "Message Name"="HH_Motor_On", "Message Queue in"=w4) -> ("error out"=w13:errorcluster, "Message Queue out"=w14:T4)  [unwired: 7 in]
  n4 = while {
    tunnel: w14 -> [w47]
    tunnel: [w43] -> w6
    tunnel: w13 -> [w41]
    tunnel: [w38] -> w5
    shift-right: [w34] -> w10
    shift-left: "?" -> [w35]
    tunnel: w8 -> [w33]
    tunnel: [w29] -> w7
    shift-right: [w20] -> w1
    shift-left: "Data in" -> [w22]
    tunnel: "AllControls In" -> [w21]
    stop <- w23 stop-if-true
    n5 = Wait (ms)(milliseconds to wait=u32 1 ("等待时间（毫秒）")) -> ()  [unwired: 1 out]
    n6 = call "AMC Read Next Message.vi"("error in (no error)"=w41, "timeout (1ms)"=100, "Message Queue in"=w47) -> ("error out"=w40:errorcluster, "Message Value"=w31:string, "Message Name"=w45:string, "Message Queue out"=w46:T4)  [unwired: 1 in, 4 out]
    n7 = case shown="\"Inlet_Blockage_Calibration\"" w45 {
      selector: w45 -> [_ w64 w102 w153 w259 w322 w364 w417 w467 w528 w579 w661]
      tunnel: w46 -> [w51 w71 w108 w162 w267 w332 w389 w424 w477 w535 w586 w669]
      tunnel: [w51 w71 w108 w162 w267 w332 w386 w424 w477 w535 w586 w669] -> w44
      tunnel: w40 -> [w50 _ w107 _ w266 _ w378 _ _ _ _ _]
      tunnel: [w50 w70 w106 w161 w265 w331 w376 w423 w476 w534 w585 w668] -> w39
      tunnel: [_ w58 _ w142 w251 w318 w380 w412 w463 w526 w574 TRUE] -> w24
      tunnel: w35 -> [w49 w56 w100 w158 w254 w328 w379 w410 w473 w523 w572 w666]
      tunnel: [w49 w56 w100 w157 w263 w327 w388 w410 w472 w523 w572 w665] -> w34
      tunnel: w31 -> [_ w69 w105 w160 w264 w330 w390 w422 w475 w533 w584 w667]
      tunnel: [_ w64 w102 w153 w259 w322 w364 w417 w467 w528 w579 w661] -> w30
      tunnel: w33 -> [_ _ _ _ _ _ _ _ _ _ _ _]
      tunnel: [_ "HH_Wait_for_X_sec_for_motor_speed_to_stabilise" "HH_get_and_check_DDM_parameter" "HH_Get_and_check_tester_Parameter" w250 w313 w381 "HH_Get_inlet_blockage_calibration(E)" w454 w508 "HH_Read_and_check_calibration" w659] -> w32
      tunnel: [_ w59 _ w143 w250 w313 w381 w413 w454 w527 w575 w659] -> w29
      tunnel: w22 -> [w48 w55 w94 w140 w243 w317 w360 w409 w451 w522 w571 w645]
      tunnel: w21 -> [_ _ _ _ w232 w302 w361 _ w447 w510 w559 w632]
      tunnel: [w48 w52 w94 w136 w242 w314 w362 w406 w448 w518 w570 w640] -> w20
      frame "假", Default {
      }
      frame "HH_Motor_On" {
        n8 = Unbundle By Name(w55) -> ("Table"=w63:string[][], "daemon reference"=w68:refnum<k5>, "Config"=w61:string[][])
        n9 = call "Select_Table_Vaule Enable_Disable.vi"("Action"=w64, "Table"=w63) -> ("Enable"=w65:bool)  [unwired: 8 in, 1 out]
        n10 = case shown="True" w65 {
          tunnel: w68 -> [w75 w93]
          tunnel: [TRUE w83] -> _
          tunnel: [w75 w87] -> w54
          tunnel: ["" ("response") w78] -> w57
          tunnel: w64 -> [_ w86]
          tunnel: w63 -> [_ w85]
          tunnel: w61 -> [_ w82]
          tunnel: "High_Power_High_Restriction_Drive_Mode" -> [_ w81]
          tunnel: [_ w80] -> w53
          tunnel: [_ w79] -> _
          tunnel: [_ w78] -> _
          tunnel: [_ w77] -> _
          frame False {
          }
          frame True {
            (unwired) "B2" ("Power Mode")
            w92 = "UIdisplay" ("Process (\"\" - local)")
            n11 = call "Index_Config.vi"("Action"=w81, "config"=w82) -> ("data"=w79:string)  [unwired: 9 in]
            n12 = call "drive_motor.vi"("Power Mode"=w79, "daemon reference in"=w93) -> ("error out"=w80:errorcluster, "response"=w78:string, "daemon reference out"=w87:refnum<k5>)  [unwired: 6 in, 1 out]
            n13 = call "Select_Table_Vaule.vi"("Vaule"=w78, "Action"=w86, "Table"=w85) -> ("Result"=w83:bool, "vaule"=w84:string[])  [unwired: 7 in]
            n14 = Append True/False String(1:w83, 2:"FAIL" ("真字符串"), 3:"PASS" ("真字符串")) -> (0:w77:string)  [unwired: 1 in]
            n15 = Build Array (concatenate)(w84, w78, w77) -> (w91:string[])
            n16 = Flatten To XML(anything=w91) -> (xml string=w90:string)
            n17 = call "AMC Send Local Message.vi"("Process (\"\" - local)"=w92, "Message Value"=w90, "Message Name"=w92) -> ()  [unwired: 7 in, 2 out]
          }
        }
        n18 = call <vilib>:"Space Constant.vi"() -> ("String"=w67:string)
        n19 = Concatenate Strings(w64, w67, w57) -> (w66:string)
        n20 = Bundle By Name(cluster=w55, "daemon reference"=w54) -> (w52:T1)
        n21 = call "LogStatus.vi"("error in (no error)"=w53, "last message"=w69, "message"=w66) -> ("error  out"=w70:errorcluster)  [unwired: 8 in]
        n22 = case shown="Error" w53 {
          tunnel: [_ TRUE] -> w58
          tunnel: [_ "Error"] -> w59
          frame No Error {
          }
          frame Error {
          }
        }
      }
      frame "HH_Wait_for_X_sec_for_motor_speed_to_stabilise" {
        (unwired) "10" ("替换字符串(\"\")")
        # "来之Config"
        n23 = Unbundle By Name(w94) -> ("Config"=w99:string[][])
        n24 = call "Index_Config.vi"("Action"="High_Power_High_Restriction_Stabilisation_Time" ("替换字符串(\"\")"), "config"=w99) -> ("data"=w97:string)  [unwired: 9 in]
        n25 = Get Date/Time In Seconds() -> (seconds since 1Jan1904=w96:timestamp)
        n26 = Fract/Exp String To Number(string=w97) -> (number=w95:dbl)  [unwired: 3 in, 1 out]
        n27 = while {
          tunnel: w96 -> [w115]
          tunnel: w95 -> [w112]
          tunnel: [w111] -> _
          stop <- w111 stop-if-true
          n28 = Get Date/Time In Seconds() -> (seconds since 1Jan1904=w116:timestamp)
          n29 = Subtract(x=w116, y=w115) -> (x-y=w114:dbl)
          n30 = call "6-AlarmStatus.vi"("Step"=enum16{"Initial", "Write", "Read"}."Read") -> ("AlarmValue Out"=w119:bool[])  [unwired: 9 in, 1 out]
          n31 = Greater Or Equal?(x=w114, y=w112) -> (x >= y?=w113:bool)
          n32 = call "Stop.vi"("Step"=enum16{"Initial", "Write", "Read"}."Read") -> ("Stop Out"=w117:bool)  [unwired: 9 in, 1 out]
          n33 = call "Exit.vi"("Step"=enum16{"Initial", "Write", "Read"}."Read" ("step")) -> ("Exit Out"=w121:bool)  [unwired: 9 in, 1 out]
          n34 = Or Array Elements(Boolean array=w119) -> (logical OR=w118:bool)
          n35 = Compound Arithmetic op=OR(w113, w117, w121, w118) -> (w111:bool)
          n36 = Wait (ms)(milliseconds to wait=u32 1 ("等待时间（毫秒）")) -> ()  [unwired: 1 out]
        }
        n37 = Search and Replace String(input string=w102, search string="X" ("搜索字符串"), replace string=w97) -> (result string=w103:string)  [unwired: 5 in, 3 out]
        n38 = call "LogStatus.vi"("error in (no error)"=w107, "last message"=w105, "message"=w103) -> ("error  out"=w106:errorcluster)  [unwired: 8 in]
      }
      frame "HH_get_and_check_DDM_parameter" {
        n39 = Unbundle By Name(w140) -> ("Table"=w152:string[][], "daemon reference"=w159:refnum<k5>, "Config"=w150:string[][])
        n40 = call "Select_Table_Vaule Enable_Disable.vi"("Action"=w153, "Table"=w152) -> ("Enable"=w151:bool)  [unwired: 8 in, 1 out]
        n41 = case shown="False" w151 {
          tunnel: w159 -> [w168 w194]
          tunnel: [w168 w193] -> w137
          tunnel: [w165 w185] -> w154
          tunnel: w153 -> [_ w190]
          tunnel: w152 -> [_ w195]
          tunnel: w150 -> [_ _]
          tunnel: [_ w179] -> w148
          tunnel: [_ w192] -> w147
          tunnel: [_ w183] -> w139
          tunnel: T6[] ["voltage", "current", "power", "speed", "measured_power", "pressure"] ("Parameter") -> [_ w178]
          tunnel: [w166 w171] -> w138
          tunnel: [w166 w169] -> w129
          frame False {
            w165 = "Skip" ("software string")
            n42 = Initialize Array(w165, 6 ("维数大小")) -> (w166:string[])
          }
          frame True {
            w184 = string[] ["HH_DDM_voltage", "HH_DDM_current", "HH_DDM_power", "HH_DDM_speed", "HH_DDM_measured_power", "HH_DDM_pressure"]
            n43 = for {
              tunnel: [w201] -> w176 mode=indexing
              tunnel: [w200] -> w183
              tunnel: [w196] -> w180 mode=indexing
              tunnel: w178 -> [w198] mode=indexing
              shift-right: [w202] -> w193
              shift-left: w194 -> [w203]
              n44 = Build Array(w198) -> (w197:T6[])
              n45 = call "get_parameter.vi"("Parameter"=w197, "daemon reference in"=w203) -> ("error out"=w200:errorcluster, "response"=w201:string, "values"=w199:dbl[], "daemon reference out"=w202:refnum<k5>)  [unwired: 5 in, 1 out]
              n46 = Index Array(array=w199) -> (element=w196:dbl)  [unwired: 1 in]
            }
            n47 = in-place {
              w208 = 1000.0
              n48 = in-place-array #1(w180, 3, 5) -> (w207:dbl, w204:dbl)
              n49 = Divide(x=w207, y=w208) -> (x/y=w206:dbl)
              n50 = Divide(x=w204, y=w208) -> (x/y=w205:dbl)
              n51 = in-place-array #1(w206, w205) -> (w179:dbl[])  [unwired: 2 out]
            }
            n52 = Array To Spreadsheet String(delimiter (Tab)=",", array=w176, 3:"" ("format string")) -> (spreadsheet string=w177:string)
            n53 = Number To Fractional String(number=w179) -> (F-format string=w171:string[])  [unwired: 3 in]
            n54 = Interleave 1D Arrays(w184, w171) -> (w188:string[])
            n55 = Build Array (concatenate)(w177, w171) -> (w189:string[])
            n56 = Array To Spreadsheet String(delimiter (Tab)=";" ("格式字符串"), array=w188, 3:"" ("格式字符串")) -> (spreadsheet string=w185:string)
            n57 = Build Array (concatenate)(w190, w184) -> (w191:string[])
            n58 = for {
              tunnel: w195 -> [w215]
              tunnel: w189 -> [w213] mode=indexing
              tunnel: w191 -> [w212] mode=indexing
              tunnel: [w211] -> w192 mode=indexing
              tunnel: [w209] -> w170 mode=indexing
              w220 = "UIdisplay" ("Process (\"\" - local)")
              n59 = call "Select_Table_Vaule.vi"("Boolean"=TRUE, "Vaule"=w213, "Action"=w212, "Table"=w215) -> ("Result"=w211:bool, "vaule"=w214:string[])  [unwired: 6 in]
              n60 = Append True/False String(1:w211, 2:"FAIL" ("真字符串"), 3:"PASS" ("真字符串")) -> (0:w209:string)  [unwired: 1 in]
              n61 = Build Array (concatenate)(w214, w213, w209) -> (w219:string[])
              n62 = Flatten To XML(anything=w219) -> (xml string=w218:string)
              n63 = call "AMC Send Local Message.vi"("Process (\"\" - local)"=w220, "Message Value"=w218, "Message Name"=w220) -> ()  [unwired: 7 in, 2 out]
            }
            n64 = Delete From Array(array=w170, length=1 ("长度"), index=0 ("索引")) -> (array with subset deleted=w169:string[])  [unwired: 1 out]
          }
        }
        n65 = call <vilib>:"Space Constant.vi"() -> ("String"=w156:string)
        n66 = Concatenate Strings(w153, w156, w154) -> (w155:string)
        n67 = Index Array(array=w138) -> (element #1=w135:string, element #2=w134:string, element #3=w133:string, element #4=w131:string, element #5=w132:string, element #6=w130:string)  [unwired: 6 in]
        n68 = Index Array(array=w129) -> (element #1=w128:string, element #2=w127:string, element #3=w126:string, element #4=w125:string, element #5=w124:string, element #6=w123:string)  [unwired: 6 in]
        n69 = Bundle By Name(cluster=w140, "daemon reference"=w137, "HH.HH - DDM Parameter - Voltage"=w135, "HH.HH - DDM Parameter - Current"=w134, "HH.HH - DDM Parameter - Power"=w133, "HH.HH - DDM Parameter - Measured Power"=w132, "HH.HH - DDM Parameter - Speed"=w131, "HH.HH - DDM Parameter - Pressure"=w130, "HH_Status.HH - DDM Parameter - Voltage"=w128, "HH_Status.HH - DDM Parameter - Current"=w127, "HH_Status.HH - DDM Parameter - Power"=w126, "HH_Status.HH - DDM Parameter - Measured Power"=w125, "HH_Status.HH - DDM Parameter - Speed"=w124, "HH_Status.HH - DDM Parameter - Pressure"=w123) -> (w136:T1)
        n70 = Delete From Array(array=w147, length=1 ("长度"), index=0 ("索引")) -> (array with subset deleted=w146:bool[])  [unwired: 1 out]
        n71 = call "LogStatus.vi"("error in (no error)"=w139, "last message"=w160, "message"=w155) -> ("error  out"=w161:errorcluster)  [unwired: 8 in]
        n72 = Bundle By Name(cluster=w158, "Task_Detect_Calib.HH.DDM_Parameter"=w148, "Task_Detect_Calib.HH.DDM_Parameter_status"=w146) -> (w157:T3)
        n73 = case shown="Error" w139 {
          tunnel: [_ TRUE] -> w142
          tunnel: [_ "Error"] -> w143
          frame No Error {
          }
          frame Error {
          }
        }
      }
      frame "HH_Get_and_check_tester_Parameter" {
        n74 = Unbundle By Name(w254) -> ("Task_Detect_Calib.HH.DDM_Parameter"=w245:dbl[])
        n75 = Unbundle By Name(w243) -> ("Table"=w244:string[][])
        n76 = call "Select_Table_Vaule Enable_Disable.vi"("Action"=w259, "Table"=w244) -> ("Enable"=w258:bool)  [unwired: 8 in, 1 out]
        n77 = case shown="False" w258 {
          tunnel: [w268 w279] -> w260
          tunnel: w259 -> [_ w285]
          tunnel: w244 -> [_ w288]
          tunnel: [_ w276] -> w257
          tunnel: [_ w287] -> w249
          tunnel: w245 -> [_ w277]
          tunnel: [w269 w272] -> w241
          tunnel: [w269 w271] -> w225
          frame False {
            w268 = "Skip" ("software string")
            n78 = Initialize Array(w268, 4 ("维数大小")) -> (w269:string[])
          }
          frame True {
            w278 = string[] ["HH_Tester_Voltage", "HH_Tester_Current", "HH_Tester_Power", "HH_DDM_Real_Power"]
            n79 = call "Task_Detect_Calibration_Calculate_Tester_Parameter.vi"("DDM Parameter"=w277) -> ("Calculate Tester Parameter"=w276:dbl[])  [unwired: 10 in]
            n80 = Number To Fractional String(number=w276) -> (F-format string=w272:string[])  [unwired: 3 in]
            n81 = Interleave 1D Arrays(w278, w272) -> (w282:string[])
            n82 = Array To Spreadsheet String(delimiter (Tab)=";" ("格式字符串"), array=w282, 3:"" ("格式字符串")) -> (spreadsheet string=w279:string)
            n83 = Build Array (concatenate)(w285, w278) -> (w286:string[])
            n84 = Build Array (concatenate)("", w272) -> (w284:string[])
            n85 = for {
              tunnel: w288 -> [w294]
              tunnel: w284 -> [w292] mode=indexing
              tunnel: w286 -> [w291] mode=indexing
              tunnel: [w290] -> w287 mode=indexing
              tunnel: [w289] -> w273 mode=indexing
              w299 = "UIdisplay" ("Process (\"\" - local)")
              n86 = call "Select_Table_Vaule.vi"("Vaule"=w292, "Action"=w291, "Table"=w294) -> ("Result"=w290:bool, "vaule"=w293:string[])  [unwired: 7 in]
              n87 = Append True/False String(1:w290, 2:"FAIL" ("真字符串"), 3:"PASS" ("真字符串")) -> (0:w289:string)  [unwired: 1 in]
              n88 = Build Array (concatenate)(w293, w292, w289) -> (w298:string[])
              n89 = Flatten To XML(anything=w298) -> (xml string=w297:string)
              n90 = call "AMC Send Local Message.vi"("Process (\"\" - local)"=w299, "Message Value"=w297, "Message Name"=w299) -> ()  [unwired: 7 in, 2 out]
            }
            n91 = Delete From Array(array=w273, length=1 ("长度"), index=0 ("索引")) -> (array with subset deleted=w271:string[])  [unwired: 1 out]
          }
        }
        n92 = Unbundle By Name(w232) -> ("MES bool"=w236:refnum<vi>)
        n93 = call "HD_Config.vi"("Step"=enum16{"Initial", "Write", "Read"}."Read") -> ("HD Config out"=w237:T5)  [unwired: 9 in, 1 out]
        n94 = call <vilib>:"Space Constant.vi"() -> ("String"=w262:string)
        n95 = Unbundle By Name(w237) -> ("Fail_resume_mode"=w235:bool)
        n96 = property class="Bool (严格)"(reference=w236) -> ("Value"=w234:bool)  [unwired: 1 in, 2 out]
        n97 = Not(x=w234) -> (.not. x?=w233:bool)
        n98 = Concatenate Strings(w259, w262, w260) -> (w261:string)
        n99 = Or(x=w235, y=w233) -> (x .or. y?=w238:bool)
        n100 = Index Array(array=w241) -> (element #1=w229:string, element #2=w228:string, element #3=w227:string, element #4=w226:string)  [unwired: 4 in]
        n101 = Index Array(array=w225) -> (element #1=w224:string, element #2=w223:string, element #3=w222:string, element #4=w221:string)  [unwired: 4 in]
        n102 = Unbundle By Name(w254) -> ("Task_Detect_Calib.HH.DDM_Parameter_status"=w253:bool[])
        n103 = Bundle By Name(cluster=w243, "HH.HH - Tester Parameter - Voltage"=w229, "HH.HH - Tester Parameter - Current"=w228, "HH.HH - Tester Parameter - Power"=w227, "HH.HH - DDM Real Power"=w226, "HH_Status.HH - Tester Parameter - Voltage"=w224, "HH_Status.HH - Tester Parameter - Current"=w223, "HH_Status.HH - Tester Parameter - Power"=w222, "HH_Status.HH - DDM Real Power"=w221) -> (w242:T1)
        n104 = Delete From Array(array=w249, length=1 ("长度"), index=0 ("索引")) -> (array with subset deleted=w248:bool[])  [unwired: 1 out]
        n105 = Build Array (concatenate)(w253, w248) -> (w252:bool[])
        n106 = call "LogStatus.vi"("error in (no error)"=w266, "last message"=w264, "message"=w261) -> ("error  out"=w265:errorcluster)  [unwired: 8 in]
        n107 = And Array Elements(Boolean array=w252) -> (logical AND=w231:bool)
        n108 = Select(t=TRUE, s=w238, f=w231) -> (s? t:f=w230:bool)
        n109 = Bundle By Name(cluster=w254, "Task_Detect_Calib.HH.Get_Tester_Parameter"=w257, "Task_Detect_Calib.HH.Get_Tester_Parameter_status"=w248) -> (w263:T3)
        n110 = Select(t="Calibrate_task_detect-HH(D)", s=w230, f="Finalization_NG_unit") -> (s? t:f=w250:string)
        n111 = Not(x=w230) -> (.not. x?=w251:bool)
      }
      frame "Calibrate_task_detect-HH(D)" {
        n112 = Unbundle By Name(w317) -> ("Table"=w321:string[][], "daemon reference"=w329:refnum<k5>, "Config"=w320:string[][])
        n113 = call "Select_Table_Vaule Enable_Disable.vi"("Action"=w322, "Table"=w321) -> ("Enable"=w323:bool)  [unwired: 8 in, 1 out]
        n114 = case shown="False" w323 {
          tunnel: w329 -> [w341 w359]
          tunnel: [TRUE w345] -> _
          tunnel: [w341 w353] -> w315
          tunnel: [w340 w344] -> w324
          tunnel: w322 -> [_ w352]
          tunnel: w321 -> [_ w351]
          tunnel: w320 -> [_ _]
          tunnel: [_ w347] -> w319
          tunnel: [_ w346] -> w316
          tunnel: [_ w345] -> w304
          tunnel: [w340 w344] -> w301
          tunnel: [w340 w343] -> w300
          frame False {
            w340 = "Skip" ("response")
          }
          frame True {
            w358 = "UIdisplay" ("Process (\"\" - local)")
            n115 = call "set_task_detect.vi"("Action"=0, "Test Point"=task_detect_test_point."HH", "daemon reference in"=w359) -> ("error out"=w346:errorcluster, "response"=w344:string, "daemon reference out"=w353:refnum<k5>)  [unwired: 5 in, 1 out]
            n116 = call "时间延迟4"("error in (no error)"=w346) -> ()  [unwired: 10 in, 1 out]
            n117 = Fract/Exp String To Number(string=w344) -> (number=w347:dbl)  [unwired: 3 in, 1 out]
            n118 = call "Select_Table_Vaule.vi"("Vaule"=w344, "Action"=w352, "Table"=w351) -> ("Result"=w345:bool, "vaule"=w350:string[])  [unwired: 7 in]
            n119 = Append True/False String(1:w345, 2:"FAIL" ("真字符串"), 3:"PASS" ("真字符串")) -> (0:w343:string)  [unwired: 1 in]
            n120 = Build Array (concatenate)(w350, w344, w343) -> (w357:string[])
            n121 = Flatten To XML(anything=w357) -> (xml string=w356:string)
            n122 = call "AMC Send Local Message.vi"("Process (\"\" - local)"=w358, "Message Value"=w356, "Message Name"=w358) -> ()  [unwired: 7 in, 2 out]
          }
        }
        n123 = call <vilib>:"Space Constant.vi"() -> ("String"=w326:string)
        n124 = Concatenate Strings(w322, w326, w324) -> (w325:string)
        n125 = Unbundle By Name(w302) -> ("MES bool"=w310:refnum<vi>)
        n126 = call "HD_Config.vi"("Step"=enum16{"Initial", "Write", "Read"}."Read") -> ("HD Config out"=w311:T5)  [unwired: 9 in, 1 out]
        n127 = Unbundle By Name(w311) -> ("Fail_resume_mode"=w309:bool)
        n128 = property class="Bool (严格)"(reference=w310) -> ("Value"=w308:bool)  [unwired: 1 in, 2 out]
        n129 = Bundle By Name(cluster=w317, "HH_Status.HH - Calibrate Task Detect HH"=w300, "HH.HH - Calibrate Task Detect HH"=w301, "daemon reference"=w315) -> (w314:T1)
        n130 = Not(x=w308) -> (.not. x?=w307:bool)
        n131 = Or(x=w309, y=w307) -> (x .or. y?=w312:bool)
        n132 = Select(t=TRUE, s=w312, f=w304) -> (s? t:f=w303:bool)
        n133 = call "LogStatus.vi"("error in (no error)"=w316, "last message"=w330, "message"=w325) -> ("error  out"=w331:errorcluster)  [unwired: 8 in]
        n134 = Bundle By Name(cluster=w328, "Task_Detect_Calib.HH.Set_task_detect_D"=w319, "Task_Detect_Calib.HH.Set_task_detect_D_Status"=w304) -> (w327:T3)
        n135 = case shown="No Error" w316 {
          tunnel: [w334 TRUE] -> w318
          tunnel: [w336 "Error"] -> w313
          tunnel: w303 -> [w333 _]
          frame No Error {
            n136 = Not(x=w333) -> (.not. x?=w334:bool)
            n137 = Select(t="Inlet_Blockage_Calibration", s=w333, f="Finalization_NG_unit") -> (s? t:f=w336:string)
          }
          frame Error {
          }
        }
      }
      frame "Inlet_Blockage_Calibration" {
        w370 = "UIdisplay" ("Process (\"\" - local)")
        n138 = Unbundle By Name(w360) -> ("Table"=w365:string[][])
        n139 = call "Select_Table_Vaule Enable_Disable.vi"("Action"=w364, "Table"=w365) -> ("Enable"=w363:bool, "vaule"=w367:string[])  [unwired: 8 in]
        n140 = call "LogStatus.vi"("error in (no error)"=w378, "last message"=w390, "message"=w364) -> ("error  out"=w377:errorcluster)  [unwired: 8 in]
        n141 = case shown="True" w363 {
          tunnel: w389 -> [w394 w405]
          tunnel: [w395 w404] -> w388
          tunnel: [w394 w403] -> w387
          tunnel: ["HH_Motor_Stop" w402] -> w381
          tunnel: w379 -> [w395 w401]
          tunnel: w377 -> [w393 w400]
          tunnel: [w393 w399] -> w376
          tunnel: [w391 w398] -> w362
          tunnel: w360 -> [w391 w397]
          tunnel: w361 -> [_ w396]
          frame False {
          }
          frame True {
            n142 = call "5.0.5_Inlet_Blockage_Calibration.vi"("Data in"=w397, "error in (no error)"=w400, "AllControls In"=w396, 10:w401, "Message Queue out"=w405) -> ("error out"=w399:errorcluster, "Flow"=w402:string, "Data"=w404:T3, "Message Queue Out"=w403:T4, "Data out"=w398:T1)  [unwired: 2 in]
          }
        }
        n143 = Select(t="Enable" ("元素"), s=w363, f="Disable" ("元素")) -> (s? t:f=w366:string)
        n144 = Append True/False String(1:w363, 2:"FAIL" ("真字符串"), 3:"PASS" ("真字符串")) -> (0:w375:string)  [unwired: 1 in]
        n145 = Build Array (concatenate)(w367, w366, w375) -> (w373:string[])
        n146 = Flatten To XML(anything=w373) -> (xml string=w374:string)
        n147 = call "AMC Send Local Message.vi"("Process (\"\" - local)"=w370, "Message Value"=w374, "Message Name"=w370) -> ()  [unwired: 7 in, 2 out]
        n148 = Flush Queue(queue=w387) -> (queue out=w386:T4)  [unwired: 1 in, 2 out]
        n149 = Equal?(x=w381, y="Finalization_NG_unit") -> (x = y?=w384:bool)
        n150 = Equal?(x=w381, y="Error") -> (x = y?=w382:bool)
        n151 = Or(x=w384, y=w382) -> (x .or. y?=w380:bool)
      }
      frame "HH_Motor_Stop" {
        n152 = Unbundle By Name(w409) -> ("Table"=w416:string[][], "daemon reference"=w421:refnum<k5>, "Config"=w415:string[][])
        n153 = call "Select_Table_Vaule Enable_Disable.vi"("Action"=w417, "Table"=w416) -> ("Enable"=w418:bool)  [unwired: 8 in, 1 out]
        n154 = case shown="True" w418 {
          tunnel: w421 -> [w428 w444]
          tunnel: [TRUE w434] -> _
          tunnel: [w428 w438] -> w407
          tunnel: ["" ("response") w432] -> w411
          tunnel: w417 -> [_ w437]
          tunnel: w416 -> [_ w436]
          tunnel: w415 -> [_ _]
          tunnel: [_ w433] -> w408
          tunnel: [_ w432] -> _
          tunnel: [_ w431] -> _
          tunnel: [_ w430] -> _
          frame False {
          }
          frame True {
            w430 = "STOP" ("Power Mode")
            w443 = "UIdisplay" ("Process (\"\" - local)")
            n155 = call "drive_motor.vi"("Power Mode"=w430, "daemon reference in"=w444) -> ("error out"=w433:errorcluster, "response"=w432:string, "daemon reference out"=w438:refnum<k5>)  [unwired: 6 in, 1 out]
            n156 = call "Select_Table_Vaule.vi"("Vaule"=w432, "Action"=w437, "Table"=w436) -> ("Result"=w434:bool, "vaule"=w435:string[])  [unwired: 7 in]
            n157 = call "时间延迟2"("error in (no error)"=w433) -> ()  [unwired: 10 in, 1 out]
            n158 = Append True/False String(1:w434, 2:"FAIL" ("真字符串"), 3:"PASS" ("真字符串")) -> (0:w431:string)  [unwired: 1 in]
            n159 = Build Array (concatenate)(w435, w432, w431) -> (w442:string[])
            n160 = Flatten To XML(anything=w442) -> (xml string=w441:string)
            n161 = call "AMC Send Local Message.vi"("Process (\"\" - local)"=w443, "Message Value"=w441, "Message Name"=w443) -> ()  [unwired: 7 in, 2 out]
          }
        }
        n162 = call <vilib>:"Space Constant.vi"() -> ("String"=w420:string)
        n163 = Concatenate Strings(w417, w420, w411) -> (w419:string)
        n164 = Bundle By Name(cluster=w409, "daemon reference"=w407) -> (w406:T1)
        n165 = call "LogStatus.vi"("error in (no error)"=w408, "last message"=w422, "message"=w419) -> ("error  out"=w423:errorcluster)  [unwired: 8 in]
        n166 = case shown="Error" w408 {
          tunnel: [_ TRUE] -> w412
          tunnel: [_ "Error"] -> w413
          frame No Error {
          }
          frame Error {
          }
        }
      }
      frame "HH_Get_inlet_blockage_calibration(E)" {
        n167 = Unbundle By Name(w451) -> ("Table"=w466:string[][], "daemon reference"=w474:refnum<k5>, "Config"=w465:string[][])
        n168 = call "Select_Table_Vaule Enable_Disable.vi"("Action"=w467, "Table"=w466) -> ("Enable"=w468:bool)  [unwired: 8 in, 1 out]
        n169 = case shown="False" w468 {
          tunnel: w474 -> [w486 w507]
          tunnel: [TRUE w492] -> _
          tunnel: [w486 w501] -> w449
          tunnel: [w485 w491] -> w469
          tunnel: w467 -> [_ w500]
          tunnel: w466 -> [_ w499]
          tunnel: w465 -> [_ _]
          tunnel: [_ w493] -> w464
          tunnel: [_ w495] -> w450
          tunnel: [_ w492] -> w452
          tunnel: [w485 w490] -> w445
          tunnel: [w485 w489] -> w446
          frame False {
            w485 = "Skip" ("response")
          }
          frame True {
            w506 = "UIdisplay" ("Process (\"\" - local)")
            n170 = call "get_calibration.vi"("Calibration"=T8[] ["eol_inlet_blockage"], "daemon reference in"=w507) -> ("error out"=w495:errorcluster, "response"=w496:string, "daemon reference out"=w501:refnum<k5>)  [unwired: 5 in, 2 out]
            n171 = Fract/Exp String To Number(string=w496) -> (number=w488:dbl)  [unwired: 3 in, 1 out]
            n172 = Divide(x=w488, y=1000.0) -> (x/y=w493:dbl)
            n173 = Number To Fractional String(number=w488) -> (F-format string=w489:string)  [unwired: 3 in]
            n174 = Number To Fractional String(number=w488) -> (F-format string=w491:string)  [unwired: 3 in]
            n175 = call "Select_Table_Vaule.vi"("Vaule"=w491, "Action"=w500, "Table"=w499) -> ("Result"=w492:bool, "vaule"=w498:string[])  [unwired: 7 in]
            n176 = Append True/False String(1:w492, 2:"FAIL" ("真字符串"), 3:"PASS" ("真字符串")) -> (0:w490:string)  [unwired: 1 in]
            n177 = Build Array (concatenate)(w498, w491, w490) -> (w505:string[])
            n178 = Flatten To XML(anything=w505) -> (xml string=w504:string)
            n179 = call "AMC Send Local Message.vi"("Process (\"\" - local)"=w506, "Message Value"=w504, "Message Name"=w506) -> ()  [unwired: 7 in, 2 out]
          }
        }
        n180 = call <vilib>:"Space Constant.vi"() -> ("String"=w471:string)
        n181 = Concatenate Strings(w467, w471, w469) -> (w470:string)
        n182 = Unbundle By Name(w447) -> ("MES bool"=w459:refnum<vi>)
        n183 = call "HD_Config.vi"("Step"=enum16{"Initial", "Write", "Read"}."Read") -> ("HD Config out"=w458:T5)  [unwired: 9 in, 1 out]
        n184 = Unbundle By Name(w458) -> ("Fail_resume_mode"=w460:bool)
        n185 = property class="Bool (严格)"(reference=w459) -> ("Value"=w461:bool)  [unwired: 1 in, 2 out]
        n186 = Not(x=w461) -> (.not. x?=w462:bool)
        n187 = Or(x=w460, y=w462) -> (x .or. y?=w457:bool)
        n188 = Select(t=TRUE, s=w457, f=w452) -> (s? t:f=w453:bool)
        n189 = Bundle By Name(cluster=w451, "Inlet Blockage Calibration_Status.Calibration Inlet Blockage_E"=w445, "daemon reference"=w449, "Inlet Blockage Calibration.Calibration Inlet Blockage_E"=w446) -> (w448:T1)
        n190 = case shown="No Error" w450 {
          tunnel: [w479 TRUE] -> w463
          tunnel: [w481 "Error"] -> w454
          tunnel: w453 -> [w478 _]
          frame No Error {
            n191 = Not(x=w478) -> (.not. x?=w479:bool)
            n192 = Select(t="HH_Set_ambient_temperature_to_DDM_ after_task_detect", s=w478, f="Finalization_NG_unit") -> (s? t:f=w481:string)
          }
          frame Error {
          }
        }
        n193 = Bundle By Name(cluster=w473, "Task_Detect_Calib.Get_eol_inlet_blockage_E"=w464, "Task_Detect_Calib.Get_eol_inlet_blockage_E_Status"=w452) -> (w472:T3)
        n194 = call "LogStatus.vi"("error in (no error)"=w450, "last message"=w475, "message"=w470) -> ("error  out"=w476:errorcluster)  [unwired: 8 in]
      }
      frame "HH_Set_ambient_temperature_to_DDM_ after_task_detect" {
        w508 = "HH_Save_calibration"
        n195 = Unbundle By Name(w523) -> ("Task_Detect_Calib.calibrated temp"=w519:dbl)
        n196 = Unbundle By Name(w522) -> ("Table"=w525:string[][], "daemon reference"=w524:refnum<k5>)
        n197 = call "Select_Table_Vaule Enable_Disable.vi"("Action"=w528, "Table"=w525) -> ("Enable"=w529:bool)  [unwired: 8 in, 1 out]
        n198 = case shown="True" w529 {
          tunnel: w524 -> [w539 w546]
          tunnel: [TRUE w549] -> _
          tunnel: [w539 w544] -> w521
          tunnel: ["" ("response") w543] -> w530
          tunnel: w528 -> [_ w552]
          tunnel: w525 -> [_ w551]
          tunnel: [_ w543] -> _
          tunnel: [_ w545] -> w520
          tunnel: w519 -> [_ w542]
          tunnel: [_ w541] -> _
          frame False {
          }
          frame True {
            w557 = "UIdisplay" ("Process (\"\" - local)")
            n199 = Build Array(w542) -> (w548:dbl[])
            n200 = call "set_calibration.vi"("values"=w548, "calibration"=T8[] ["eol_cold_bemf_temp"], "daemon reference in"=w546) -> ("error out"=w545:errorcluster, "response"=w543:string, "daemon reference out"=w544:refnum<k5>)  [unwired: 5 in, 1 out]
            n201 = call "Select_Table_Vaule.vi"("Vaule"=w543, "Action"=w552, "Table"=w551) -> ("Result"=w549:bool, "vaule"=w550:string[])  [unwired: 7 in]
            n202 = Append True/False String(1:w549, 2:"FAIL" ("真字符串"), 3:"PASS" ("真字符串")) -> (0:w541:string)  [unwired: 1 in]
            n203 = Build Array (concatenate)(w550, w543, w541) -> (w556:string[])
            n204 = Flatten To XML(anything=w556) -> (xml string=w555:string)
            n205 = call "AMC Send Local Message.vi"("Process (\"\" - local)"=w557, "Message Value"=w555, "Message Name"=w557) -> ()  [unwired: 7 in, 2 out]
          }
        }
        n206 = call <vilib>:"Space Constant.vi"() -> ("String"=w532:string)
        n207 = Unbundle By Name(w510) -> ("MES bool"=w514:refnum<vi>)
        n208 = Concatenate Strings(w528, w532, w530) -> (w531:string)
        n209 = call "HD_Config.vi"("Step"=enum16{"Initial", "Write", "Read"}."Read") -> ("HD Config out"=w513:T5)  [unwired: 9 in, 1 out]
        n210 = Unbundle By Name(w513) -> ("Fail_resume_mode"=w515:bool)
        n211 = property class="Bool (严格)"(reference=w514) -> ("Value"=w516:bool)  [unwired: 1 in, 2 out]
        n212 = Not(x=w516) -> (.not. x?=w517:bool)
        n213 = Or ("或")(x=w515, y=w517) -> (x .or. y?=w512:bool)
        n214 = Select(t="HH_Read_and_check_calibration", s=w512, f=w508) -> ()  [unwired: 1 out]
        n215 = Bundle By Name(cluster=w522, "daemon reference"=w521) -> (w518:T1)
        n216 = call "LogStatus.vi"("error in (no error)"=w520, "last message"=w533, "message"=w531) -> ("error  out"=w534:errorcluster)  [unwired: 8 in]
        n217 = case shown="Error" w520 {
          tunnel: [_ TRUE] -> w526
          tunnel: [_ "Error"] -> w527
          frame No Error {
          }
          frame Error {
          }
        }
      }
      frame "HH_Save_calibration" {
        n218 = Unbundle By Name(w571) -> ("Table"=w578:string[][], "daemon reference"=w583:refnum<k5>, "Config"=w577:string[][])
        n219 = Unbundle By Name(w559) -> ("MES bool"=w564:refnum<vi>)
        n220 = call "HD_Config.vi"("Step"=enum16{"Initial", "Write", "Read"}."Read") -> ("HD Config out"=w565:T5)  [unwired: 9 in, 1 out]
        n221 = Unbundle By Name(w565) -> ("Fail_resume_mode"=w563:bool)
        n222 = property class="Bool (严格)"(reference=w564) -> ("Value"=w562:bool)  [unwired: 1 in, 2 out]
        n223 = call "Select_Table_Vaule Enable_Disable.vi"("Action"=w579, "Table"=w578) -> ("Enable"=w580:bool)  [unwired: 8 in, 1 out]
        n224 = Not(x=w562) -> (.not. x?=w561:bool)
        n225 = Or ("或")(x=w563, y=w561) -> (x .or. y?=w558:bool)
        n226 = case shown="False" w580 {
          tunnel: w583 -> [w590 w604]
          tunnel: [TRUE w596] -> _
          tunnel: [w590 w600] -> w568
          tunnel: [w589 w594] -> w573
          tunnel: w579 -> [_ w599]
          tunnel: w578 -> [_ w598]
          tunnel: w577 -> [_ _]
          tunnel: [_ w595] -> w569
          tunnel: [w589 w594] -> w567
          tunnel: [w589 w593] -> w566
          tunnel: w558 -> [_ w592]
          frame False {
            w589 = "Skip" ("response")
          }
          frame True {
            w603 = "UIdisplay" ("Process (\"\" - local)")
            n227 = case shown="True" w592 {
              tunnel: w604 -> [w613 w615]
              tunnel: [w612 w615] -> w600
              tunnel: [w611 _] -> w595
              tunnel: [w610 "Skip" ("response")] -> w594
              frame False {
                n228 = call "finalise_calibration.vi"("daemon reference in"=w613) -> ("error out"=w611:errorcluster, "response"=w610:string, "daemon reference out"=w612:refnum<k5>)  [unwired: 7 in, 1 out]
                n229 = call "时间延迟3"("error in (no error)"=w611) -> ()  [unwired: 10 in, 1 out]
              }
              frame True {
              }
            }
            n230 = call "Select_Table_Vaule.vi"("Vaule"=w594, "Action"=w599, "Table"=w598) -> ("Result"=w596:bool, "vaule"=w597:string[])  [unwired: 7 in]
            n231 = case shown="True" w592 {
              tunnel: w596 -> [w606 _]
              tunnel: [w605 "Skip" ("response")] -> w593
              frame False {
                n232 = Append True/False String(1:w606, 2:"FAIL" ("真字符串"), 3:"PASS" ("真字符串")) -> (0:w605:string)  [unwired: 1 in]
              }
              frame True {
              }
            }
            n233 = Build Array (concatenate)(w597, w594, w593) -> (w602:string[])
            n234 = Flatten To XML(anything=w602) -> (xml string=w601:string)
            n235 = call "AMC Send Local Message.vi"("Process (\"\" - local)"=w603, "Message Value"=w601, "Message Name"=w603) -> ()  [unwired: 7 in, 2 out]
          }
        }
        n236 = call <vilib>:"Space Constant.vi"() -> ("String"=w582:string)
        n237 = Concatenate Strings(w579, w582, w573) -> (w581:string)
        n238 = Bundle By Name(cluster=w571, "Inlet Blockage Calibration_Status.Finalise Calibration"=w566, "Inlet Blockage Calibration.Finalise Calibration"=w567, "daemon reference"=w568) -> (w570:T1)
        n239 = call "LogStatus.vi"("error in (no error)"=w569, "last message"=w584, "message"=w581) -> ("error  out"=w585:errorcluster)  [unwired: 8 in]
        n240 = case shown="Error" w569 {
          tunnel: [_ TRUE] -> w574
          tunnel: [_ "Error"] -> w575
          frame No Error {
          }
          frame Error {
          }
        }
      }
      frame "HH_Read_and_check_calibration" {
        n241 = Unbundle By Name(w666) -> ("Task_Detect_Calib.LL.Set_task_detect_A"=w657:dbl, "Task_Detect_Calib.HL.Set_task_detect_B"=w656:dbl, "Task_Detect_Calib.LH.Set_task_detect_C"=w655:dbl, "Task_Detect_Calib.HH.Set_task_detect_D"=w654:dbl, "Task_Detect_Calib.Get_eol_inlet_blockage_E"=w649:dbl, "Task_Detect_Calib.calibrated temp"=w651:dbl)
        n242 = Unbundle By Name(w645) -> ("Table"=w647:string[][], "daemon reference"=w646:refnum<k5>)
        n243 = Multiply(x=w649, y=1000.0) -> (x*y=w650:dbl)
        n244 = Build Array(w657, w656, w655, w654, w650, w651) -> (w642:dbl[])
        n245 = call "Select_Table_Vaule Enable_Disable.vi"("Action"=w661, "Table"=w647) -> ("Enable"=w660:bool)  [unwired: 8 in, 1 out]
        n246 = case shown="False" w660 {
          tunnel: w646 -> [w681 w709]
          tunnel: [w681 w697] -> w639
          tunnel: [w680 w703] -> w662
          tunnel: w661 -> [_ w707]
          tunnel: w647 -> [_ w710]
          tunnel: [_ w693] -> w652
          tunnel: [_ w691] -> w643
          tunnel: [w679 w690] -> w644
          tunnel: w642 -> [_ w689]
          tunnel: [_ w688] -> w641
          tunnel: [w679 w682] -> w622
          frame False {
            w680 = "Skip" ("software string")
            n247 = Initialize Array(w680, 6 ("维数大小")) -> (w679:string[])
          }
          frame True {
            w701 = T7[] [enum."LL", enum."HL", enum."LH", enum."HH"] items=["LL", "HL", "LH", "HH"]
            w702 = string[] ["HH_Get_task_detect::LL", "HH_Get_task_detect::HL", "HH_Get_task_detect::LH", "HH_Get_task_detect::HH", "HH_Get_calibration::eol_inlet_blockage", "HH_Get_calibration::eol_cold_bemf_temp"]
            n248 = for {
              tunnel: [w720] -> w696 mode=indexing
              shift-right: [w721] -> w698
              shift-left: w709 -> [w722]
              tunnel: w701 -> [w719] mode=indexing
              tunnel: [w718] -> w692
              n249 = call "get_task_detect.vi"("Test Point"=w719, "daemon reference in"=w722) -> ("error out"=w718:errorcluster, "response"=w720:string, "daemon reference out"=w721:refnum<k5>)  [unwired: 6 in, 1 out]
            }
            n250 = for {
              tunnel: T8[] ["eol_inlet_blockage", "eol_cold_bemf_temp"] ("Calibration") -> [w717] mode=indexing
              tunnel: [w714] -> w695 mode=indexing
              shift-right: [w715] -> w697
              shift-left: w698 -> [w716]
              shift-right: [w712] -> w691
              shift-left: w692 -> [w713]
              n251 = Build Array(w717) -> (w711:T8[])
              n252 = call "get_calibration.vi"("error in (no error)"=w713, "Calibration"=w711, "daemon reference in"=w716) -> ("error out"=w712:errorcluster, "response"=w714:string, "daemon reference out"=w715:refnum<k5>)  [unwired: 4 in, 2 out]
            }
            n253 = Build Array (concatenate)(w696, w695) -> (w690:string[])
            n254 = Interleave 1D Arrays(w702, w690) -> (w706:string[])
            n255 = Build Array (concatenate)("", w690) -> (w694:string[])
            n256 = Fract/Exp String To Number(string=w690) -> (number=w693:dbl[])  [unwired: 3 in, 1 out]
            n257 = Array To Spreadsheet String(delimiter (Tab)=";" ("格式字符串"), array=w706, 3:"" ("格式字符串")) -> (spreadsheet string=w703:string)
            n258 = Build Array (concatenate)(w707, w702) -> (w708:string[])
            n259 = Equal?(x=w693, y=w689) -> (x = y?=w688:bool[])
            n260 = Build Array (concatenate)(TRUE, w688) -> (w686:bool[])
            n261 = for {
              tunnel: w710 -> [w728]
              tunnel: w694 -> [w726] mode=indexing
              tunnel: w708 -> [w725] mode=indexing
              tunnel: w686 -> [w724] mode=indexing
              tunnel: [w723] -> w683 mode=indexing
              w733 = "UIdisplay" ("Process (\"\" - local)")
              n262 = call "Select_Table_Vaule.vi"("Vaule"=w726, "Action"=w725, "Table"=w728) -> ("vaule"=w727:string[])  [unwired: 7 in, 1 out]
              n263 = Append True/False String(1:w724, 2:"FAIL" ("真字符串"), 3:"PASS" ("真字符串")) -> (0:w723:string)  [unwired: 1 in]
              n264 = Build Array (concatenate)(w727, w726, w723) -> (w732:string[])
              n265 = Flatten To XML(anything=w732) -> (xml string=w731:string)
              n266 = call "AMC Send Local Message.vi"("Process (\"\" - local)"=w733, "Message Value"=w731, "Message Name"=w733) -> ()  [unwired: 7 in, 2 out]
            }
            n267 = Delete From Array(array=w683, length=1 ("长度"), index=0 ("索引")) -> (array with subset deleted=w682:string[])  [unwired: 1 out]
          }
        }
        n268 = call <vilib>:"Space Constant.vi"() -> ("String"=w664:string)
        n269 = Concatenate Strings(w661, w664, w662) -> (w663:string)
        n270 = Unbundle By Name(w632) -> ("MES bool"=w637:refnum<vi>)
        n271 = call "HD_Config.vi"("Step"=enum16{"Initial", "Write", "Read"}."Read") -> ("HD Config out"=w638:T5)  [unwired: 9 in, 1 out]
        n272 = Array To Cluster(array=w652) -> (cluster=w653:T9)
        n273 = Unbundle By Name(w638) -> ("Fail_resume_mode"=w636:bool)
        n274 = property class="Bool (严格)"(reference=w637) -> ("Value"=w635:bool)  [unwired: 1 in, 2 out]
        n275 = Index Array(array=w622) -> (element #1=w621:string, element #2=w620:string, element #3=w619:string, element #4=w618:string, element #5=w617:string, element #6=w616:string)  [unwired: 6 in]
        n276 = Index Array(array=w644) -> (element #1=w628:string, element #2=w627:string, element #3=w626:string, element #4=w625:string, element #5=w624:string, element #6=w623:string)  [unwired: 6 in]
        n277 = Not(x=w635) -> (.not. x?=w634:bool)
        n278 = Or(x=w636, y=w634) -> (x .or. y?=w629:bool)
        n279 = Bundle By Name(cluster=w645, "daemon reference"=w639, "Inlet Blockage Calibration.Get Task Detect LL"=w628, "Inlet Blockage Calibration.Get Task Detect HL"=w627, "Inlet Blockage Calibration.Get Task Detect LH"=w626, "Inlet Blockage Calibration.Get Task Detect HH"=w625, "Inlet Blockage Calibration.Calibration Inlet Blockage"=w624, "Inlet Blockage Calibration.Calibration eol cold bemf temp"=w623, "Inlet Blockage Calibration_Status.Get Task Detect LL"=w621, "Inlet Blockage Calibration_Status.Get Task Detect HL"=w620, "Inlet Blockage Calibration_Status.Get Task Detect LH"=w619, "Inlet Blockage Calibration_Status.Get Task Detect HH"=w618, "Inlet Blockage Calibration_Status.Calibration Inlet Blockage"=w617, "Inlet Blockage Calibration_Status.Calibration eol cold bemf temp"=w616) -> (w640:T1)
        n280 = call "LogStatus.vi"("error in (no error)"=w643, "last message"=w667, "message"=w663) -> ("error  out"=w668:errorcluster)  [unwired: 8 in]
        n281 = And Array Elements(Boolean array=w641) -> (logical AND=w631:bool)
        n282 = case shown="No Error" w643 {
          tunnel: [w671 "Error"] -> w659
          tunnel: w631 -> [w674 _]
          tunnel: "Finalization_NG_unit" -> [w673 _]
          tunnel: w629 -> [w670 _]
          frame No Error {
            n283 = Select(t="Finalization_good_unit", s=w674, f="Finalization_NG_unit") -> (s? t:f=w672:string)
            n284 = Select(t=w673, s=w670, f=w672) -> (s? t:f=w671:string)
          }
          frame Error {
          }
        }
        n285 = Bundle By Name(cluster=w666, "Task_Detect_Calib.Calib_vaule"=w653, "Task_Detect_Calib.HH.Read_and_check_calibration_Status"=w641) -> (w665:T3)
      }
    }
    n286 = call "6-AlarmStatus.vi"("Step"=enum16{"Initial", "Write", "Read"}."Read") -> ("AlarmValue Out"=w18:bool[])  [unwired: 9 in, 1 out]
    n287 = call "Stop.vi"("Step"=enum16{"Initial", "Write", "Read"}."Read") -> ("Stop Out"=w26:bool)  [unwired: 9 in, 1 out]
    n288 = call "Exit.vi"("Step"=enum16{"Initial", "Write", "Read"}."Read" ("step")) -> ("Exit Out"=w25:bool)  [unwired: 9 in, 1 out]
    n289 = Or Array Elements(Boolean array=w18) -> (logical OR=w17:bool)
    n290 = Compound Arithmetic op=OR(w24, w26, w25, w17) -> (w23:bool)
    n291 = call "AMC Run Step.vi"("Message Queue In"=w44, "Message Name"=w32, "Message Value"=w30, "error in (no error)"=w39, "Mli/Sig"=FALSE) -> ("Message Queue Out"=w43:T4, "error out"=w38:errorcluster)  [unwired: 13 in]
  }
  "Message Queue Out" <- w6
  "error out" <- w5
  "Data" <- w10
  "Flow" <- w7
  "Data out" <- w1
